vi "UHR-Fleezers Control (fpga) - 10.8c.vi"() -> ()   [LabVIEW 2014]
doc: "UHR-Fleezers Instrument Control Code (fpga)"
uses:
  <vilib>/eio/EIONode/EIONode.xnode
  <vilib>/eio/EIOMethodNode/EIOMethodNode.xnode
  <vilib>/rvi/DataTransferAndStorage/Container/XNode/niFpgaContainer.xnode
  <vilib>/Platform/TimedLoop/XDataNode/XDataNode.xnode
  <vilib>/Platform/TimedLoop/XDataNode/nitl_modes.ctl
  <vilib>/Platform/TimedLoop/XDataNode/XDNodeRunTimeDep.lvlib
  <vilib>/Platform/TimedLoop/XDataNode/wakeup.ctl
  <vilib>/Platform/TimedLoop/XDataNode/timing_clust.ctl
  <vilib>/addons/control/pid/fpga.llb/XNode/niFpgaPID.xnode
  <vilib>/rvi/eio/common/nirviEmuTemplateMethod_errors.vi
  <vilib>/rvi/interface/RandomDataEmulation/nirviRandomDataFpgaReadWriteTemplate.vi
panel:
  in  "Connector0/AO6":i16
  in  "Tab Control":T1(tab)=enum."Force FB"
  in  "Trap Pos to FIFO":bool
  in  "AI1 Sets to FIFO":T2={"Set 1"=TRUE, "Set 2"=TRUE, "Set 3"=FALSE}
  in  "N of AI1 Int Acq Sets":i16=2 min=1 max=3 step=1
  out "AI Late Counter":u8
  in  "ai count":u16=400
  in  "+ phase":bool
  in  "Phase count adjustment":i16
  out "Relative phase":i16
  in  "AI to FIFO":bool
  out "BD1 Frequency Out 1":u64
  out "BD1 Frequency Out 2":u64
  out "Trap Pos FIFO Timeout":u16
  out "Trap AI FIFO Timeout":u16
  in  "Trap FIFO Set Timeout":i32
  in  "Tab Control 2":T3(tab)
  out "Wiggling 2":bool
  in  "Abort wiggle 2":bool
  in  "Wiggle amp 2":u64
  in  "Wiggle freq 2 (Hz)":fxp<+/-,16,16>
  in  "Wiggle trap 2":bool
  out "Wiggling 1":bool
  in  "Abort wiggle 1":bool
  in  "Wiggle trap 1":bool
  in  "Wiggle amp 1":u64
  in  "Wiggle freq 1 (Hz)":fxp<+/-,16,16>
  in  "Swap F1 and F2":bool
  in  "Freq or Amp switch first":bool=TRUE
  in  "Cont. Scan":bool
  in  "Abort scan":bool
  in  "Cycles per step":u64
  in  "Scan BD":bool
  in  "Number of scans":u16
  in  "Scan steps":u64
  in  "Scan freq.  increment":i64
  out "Scanning":bool
  in  "Start scan":bool
  in  "OSK Bd 1":bool
  in  "Reset Bd 1":bool
  in  "RD":bool
  in  "PMODE":bool
  in  "OSK Bd 2":bool
  in  "Reset Bd 2":bool
  in  "Direct RF Box \nCommunication":bool
  in  "Data BD 2":u8 format="%08b"
  in  "Data BD 1":u8 format="%08b"
  in  "Address":u8 format="%02x"
  in  "Update Data":bool
  in  "FPGA Controls\n RF Box":bool
  in  "Number Interlace Cycles":u8=2 min=1 max=3
  in  "Interlace Off Parameters":u8=1 min=1 max=3
  in  "Interlace ON/OFF":bool
  out "DIO Relative phase":i16
  in  "Phase count adjustment (DIO)":i16
  in  "+ phase (DIO)":bool
  out "DIO Late Counter":u8
  in  "DIO count 1 (ticks)":u16=400
  in  "DIO count 2 (ticks)":u16=400
  in  "DIO count 3 (ticks)":u16=400
  out "AI2 Y Sum Set 2":i16
  out "AI2 Y Sum Set 1":i16
  in  "FB Gains Set 1":T4={"proportional gain (Kc)"=10, "integral gain (Kc*Ts/Ti)"=5, "derivative gain (Kc*Td/Ts)"=0}
  in  "FB Setpoint Set 1":i16 min=0 step=1
  in  "FB Reset Set 1":bool
  in  "FB On/Off Set 1":bool
  in  "FB Reset Set 2":bool
  in  "FB On/Off Set 2":bool
  in  "FB Setpoint Set 2":i16 min=0 step=1
  in  "FB Gains Set 2":T4={"proportional gain (Kc)"=10, "integral gain (Kc*Ts/Ti)"=5, "derivative gain (Kc*Td/Ts)"=0}
  in  "FB output range 2":cluster{"output high":i16, "output low":i16}={"output high"=3000, "output low"=0}
  in  "FB output range 1":cluster{"output high":i16, "output low":i16}={"output high"=3000, "output low"=0}
  out "Scan I":u64
  in  "Amp switch delay":u16=5
  in  "Freq switch delay":u16
  in  "BD 2 Amplitude 1":u16
  in  "BD 1 Amplitude 1":u16
  in  "BD 2 Frequency 1":u64
  in  "BD 1 Frequency 1":u64
  in  "BD 2 Amplitude 2":u16
  in  "BD 1 Amplitude 2":u16
  in  "BD 2 Frequency 2":u64
  in  "BD 1 Frequency 2":u64
  in  "BD 2 Amplitude 3":u16
  in  "BD 1 Amplitude 3":u16
  in  "BD 2 Frequency 3":u64
  in  "BD 1 Frequency 3":u64
  in  "Negate Diff?":bool
  in  "Diff FB Measurement?":bool
  in  "FB Trig Integrate":u32=1
  out "TTrig?":bool
  in  "TTrig Negate Pos":bool=TRUE
  out "Trap Pos FB Int Signal":fxp<+/-,24,9> format="%.18g"
  out "Trap Pos FB Int-Norm Signal":fxp<+/-,16,1> format="%.16g"
  in  "FPGA TTrig Thresh":i64
  in  "FPGA Trap Trig":bool
  out "Trap Pos FB Action":i64
  in  "Trap Pos. FB Offset Factor":i64
  in  "Trap Pos. FB Mult Factor":i64=2
  in  "Trap Pos. FB Range":T5={"output high"=0.999969482421875, "output low"=-1.0}
  in  "Trap Pos. FB Gains":T6={"proportional gain (Kc)"=0.0, "integral gain (Kc*Ts/Ti)"=10.0, "derivative gain (Kc*Td/Ts)"=0.0} {"proportional gain (Kc)" format="%.11g"; "integral gain (Kc*Ts/Ti)" format="%.11g"; "derivative gain (Kc*Td/Ts)" format="%.11g"}
  in  "Trap Pos. FB Reset":bool
  in  "Trap Pos FB Monitor T1 or T2":bool
  in  "AI1 X Scale":u16
  in  "Trap Pos FB Int Count":u16=100
  in  "Trap Pos FB Negate Action":bool
  out "AI1 X Set 2":fxp<+/-,16,1>
  out "AI1 X Set 1":fxp<+/-,16,1>
  in  "Trap Pos. FB SP":fxp<+/-,16,1>
  in  "Force feedback":bool
  out "TTrig Sig":i64
  out "TTrig Fin Thresh":i64
  out "Numeric":i32
  out "AO2 2":i16
  out "AO1 2":i16
  in  "1D or 2D Scan?":bool
  in  "Abort scan (MCL)":bool
  in  "MCL Scan Axis":bool
  in  "Cont. Scan (MCL)":bool
  out "Scan I (MCL)":u64
  in  "Number of scans (MCL)":u16
  out "Scanning MCL":bool
  in  "Scan steps (MCL)":u64
  in  "Cycles per step (MCL)":u64
  in  "Scan freq.  increment (MCL)":i16
  in  "Start scan (MCL)":bool
  in  "AO2":i16
  in  "AO1":i16
  out "MCL Late Counter":u8
  in  "MCL count":u32=800
  out "MCL Relative Phase":i16
  in  "Phase count adjustment (MCL)":i16
  in  "+ phase (MCL)":bool
  in  "APD Gate Operating Mode":u8 max=2 step=1
  in  "Invert APD Gate":bool
  in  "APD Gate OFF Count":u16=100
  in  "APD Gate ON Count":u16=300
  out "APD 1 Gate Late Counter":u8
  out "APD 1 Gate Relative Phase":i16
  in  "Phase count adjustment (APD 1 Gate)":i16
  in  "+ phase (APD 1 Gate)":bool
  out "APD 2 Counts 0":u32
  out "APD 2 Counts 1":u32
  out "APD 1 Counts 0":u32
  out "APD 1 Counts 1":u32
  out "APD 1 out state":bool
  in  "APD 2 AO scale factor":i16=1
  in  "APD 1 AO scale factor":i16=1
  in  "APD to FIFO":bool
  in  "APD Acq Rate Count":u32=20000000
  out "APD Acq Late Counter":u8
  out "APD Acq Relative Phase":i16
  in  "Phase Count Adjustment (APD Acq)":i16
  in  "+ phase (APD Acq)":bool
  in  "Phase count adjustment (APD 2 Gate)":i16
  out "APD 2 Gate Late Counter":u8
  out "APD 2 Gate Relative Phase":i16
  in  "+ phase (APD 2 Gate)":bool
  out "APD 2 out state":bool
  out "APD 1 Int Gate":bool
  out "APD 2 Int Gate":bool
  in  "Green Filter Flipper":bool
  out "Green FB Signals":T7
  in  "Green FB Count":u16=1200
  out "Green Late Counter":u8
  out "Green FB Relative Phase":i16
  in  "Phase count adjustment (Green FB)":i16=10
  in  "+ phase (Green FB)":bool
  out "Green FB Sum":i16
  in  "Green int current ON count adj":u16=150
  in  "Current Out":u16=30000
  in  "Green FB On/Off":bool
  in  "Green FB Setpoint":i16=250 min=0 step=1
  in  "Green FB Gains":T4={"proportional gain (Kc)"=10, "integral gain (Kc*Ts/Ti)"=5, "derivative gain (Kc*Td/Ts)"=0}
  in  "Green FB Reset":bool
  in  "Operating Mode 2":u8=2 max=2 step=1
  in  "Invert GI 2":bool
  in  "Green interlace OFF count 2":u16=900
  in  "Green interlace ON count 2":u16=300
  out "GI Late Counter 2":u8
  out "GI Relative phase 2":i16
  in  "Phase count adjustment (GI) 2":i16=20
  in  "+ phase (GI) 2":bool
  in  "Green interlace OFF count":u16=100
  out "GI Relative phase":i16
  in  "Phase count adjustment (GI)":i16
  in  "+ phase (GI)":bool
  in  "Green interlace ON count":u16=300
  out "GI Late Counter":u8
  in  "Invert GI":bool
  in  "Operating Mode":u8 max=2 step=1
  in  "Invert RI 2":bool
  in  "Invert RI":bool
  in  "Phase count adjustment (RI)":i16
  in  "+ phase (RI)":bool
  in  "RI OFF count":u16
  in  "RI ON count":u16
  in  "RI Current Out":u16
  in  "RI operating mode 2":u8
  in  "Red operating mode":u8
  out "RI late counter":u8
  out "RI relative phase":i16
  in  "Chassis2/Mod4/AO1":u16
  # "Only one of these can be on\nat a time:"
  # "Raster Scan AOD"
  # "1 (X)"
  # "2 (Y)"
  # "IR Intensity Feedback (RF BD 1)"
  # "FB Triggering Excitation Laser"
  # "AO1 (Y)"
  # "2D"
  # "1D"
  # "AO2 (X)"
  # "APD AO for aligning"
  # "Detection Loop"
  # "Green fluorescent laser digital gate interlacing loop"
  # "0 Forced ON\n1 Forced OFF\n2 Interlacing"
  # "Red fluorescent laser digital gate interlacing loop"
  # "0 Forced ON\n1 Forced OFF\n2 Interlacing"
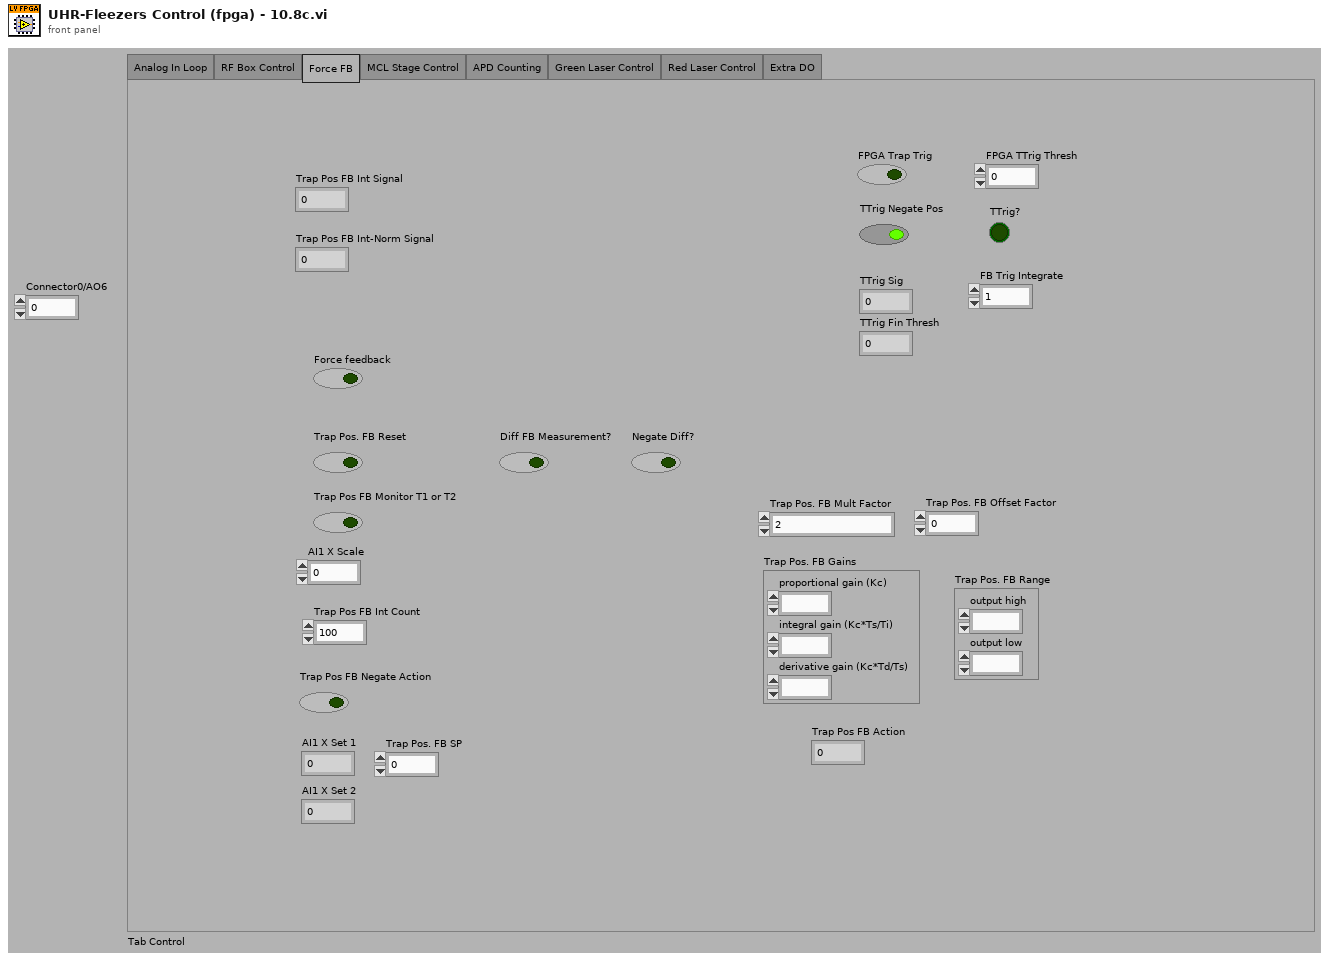
[diagram p1: front panel]
types:
  T1 = enum32{"Analog In Loop", "RF Box Control", "Force FB", "MCL Stage Control", "APD Counting", "Green Laser Control", "Red Laser Control", "Extra DO"}
  T2 = cluster{"Set 1":bool, "Set 2":bool, "Set 3":bool}
  T3 = enum32{"Controls", "Interlacing Frequency and Amplitude Values"}
  T4 = cluster{"proportional gain (Kc)":i16, "integral gain (Kc*Ts/Ti)":i16, "derivative gain (Kc*Td/Ts)":i16}
  T5 = cluster{"output high":fxp<+/-,16,1>, "output low":fxp<+/-,16,1>}
  T6 = cluster{"proportional gain (Kc)":fxp<+/-,16,8>, "integral gain (Kc*Ts/Ti)":fxp<+/-,16,8>, "derivative gain (Kc*Td/Ts)":fxp<+/-,16,8>}
  T7 = cluster{"Green FB Ch 0":i16, "Green FB Ch 1":i16, "Green FB Ch 2":i16}
  T8 = typedef "XDNodeRunTimeDep.lvlib/timing_clust.ctl" = cluster{"Expected End [f-1]":u64, "Actual End [f-1]":u64, "Finished Late? [f-1]":bool, "Expected End [i-1]":u64, "Actual End [i-1]":u64, "Finished Late? [i-1]":bool, "Expected Start [i]":u64, "Actual Start [i]":u64, "Expected Start [f]":u64, "Actual Start [f]":u64, "Source Name":string, "Structure Name":string, "Period":i64, "Deadline":i64, "Offset":i64, "Start":i64, "Priority":i32, "Timeout":i32, "Mode":T9, "Wakeup Reason":T10, "Error":errorcluster, "Source Type":string, "Secondary Source Type":string, "Global End Time":u64, "Global Start Time":u64, "Frame Duration":u64, "Iteration Duration":u64, "Assigned CPU":i32, "I/O Scan Engine Mode":u32}
  T9 = typedef "XDNodeRunTimeDep.lvlib/nitl_modes.ctl" = enum32{"No Change", "Process missed periods, maintain original phase", "Discard missed periods, maintain original phase", "Process missed periods, ignore original phase", "Discard missed periods, ignore original phase"}
  T10 = typedef "XDNodeRunTimeDep.lvlib/wakeup.ctl" = enum32{"Normal", "Aborted", "Asynchronous wakeup", "Timing source error", "Timed loop error", "Timeout"}
  T11 = cluster{"Chassis2/Mod1/AI0":void, "Chassis2/Mod1/AI1":void, "Chassis2/Mod1/AI2":void}
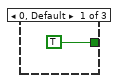
[diagram p2: hidden frame]
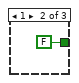
[diagram p3: hidden frame]
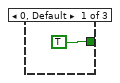
[diagram p4: hidden frame]
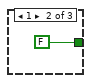
[diagram p5: hidden frame]
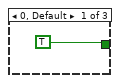
[diagram p6: hidden frame]
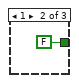
[diagram p7: hidden frame]
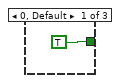
[diagram p9: hidden frame]
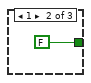
[diagram p10: hidden frame]
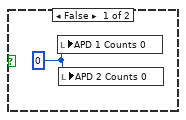
[diagram p11: hidden frame]
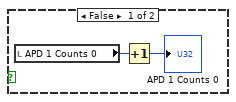
[diagram p14: hidden frame]
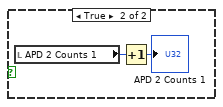
[diagram p16: hidden frame]
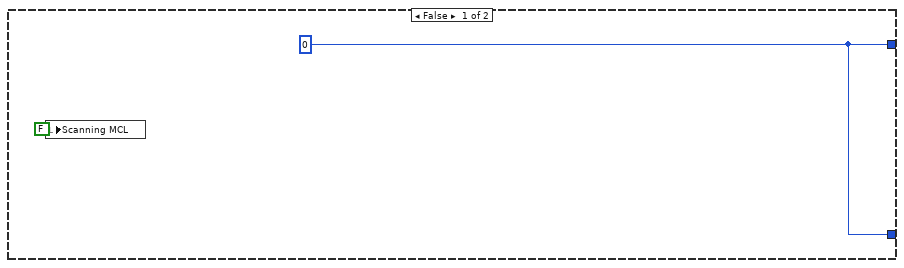
[diagram p17: hidden frame]
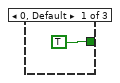
[diagram p18: hidden frame]
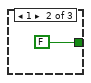
[diagram p19: hidden frame]
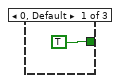
[diagram p20: hidden frame]
diagram:
  w1 = u16 0
  w4 = FALSE
  w2 = FALSE
  # "633 nm red excitation laser interlacing (DO to IA 633 nm AOM ME amp)."
  # "The APD Int Gate is here so the FPGA will do the integration only when the APD gate is \"ON\" (though we will leave the APD continuously ON now). This was added because the actual APD gating (via the hardware) was giving false signals. -KW"
  # "timing array current index"
  # "timing array"
  # "timing counter (phase adjusted here)"
  # "late counter"
  n1 = flat-sequence "FPGA initialization to do before running any of the loops" {
    tunnel: [u16 0 ("DIO count 3 (ticks)")] -> w3
    tunnel: [w10] -> _
    frame #0 {
      # "Start up expansion chassis early\nto avoid delays later"
      # "This pin controls udclk on the RF boards.\nWhen initially configuring the boards, this pin needs to be\nconfigured as a high impedance input.  Later it will be switched\nto an output."
      # "Initial setting of DIO data and \naddress to low (before reset).  \nThis needs to happen before the other\ncontrol method loops execute."
      n2 = xnode "FPGA I/O Node"("Chassis2/Mod4/AO0"=u16 0) -> ("Chassis2/Mod1/AI0"=w10)  [unwired: 2 in, 2 out]
      n3 = xnode "FPGA I/O Method Node"("Enable"=FALSE) -> ()  [unwired: 1 in, 1 out]
      n4 = xnode "FPGA I/O Node"("Connector1/DIO0"=FALSE, "Connector1/DIO1"=FALSE, "Connector1/DIO2"=FALSE, "Connector1/DIO3"=FALSE, "Connector1/DIO4"=FALSE, "Connector1/DIO5"=FALSE, "Connector1/DIO6"=FALSE, "Connector1/DIO7"=FALSE, "Connector1/DIO8"=FALSE, "Connector1/DIO9"=FALSE, "Connector1/DIO10"=FALSE, "Connector1/DIO11"=FALSE, "Connector1/DIO12"=FALSE, "Connector1/DIO13"=FALSE, "Connector1/DIO15"=FALSE, "Connector1/DIO20"=FALSE, "Connector1/DIO21"=FALSE, "Connector1/DIO22"=FALSE, "Connector1/DIO23"=FALSE, "Connector1/DIO24"=FALSE, "Connector1/DIO25"=FALSE, "Connector1/DIO26"=FALSE, "Connector1/DIO27"=FALSE, "Connector1/DIO14"=FALSE) -> ()  [unwired: 24 in, 24 out]
    }
  }
  n5 = local read "AO1"() -> (w8:i16)
  n6 = local read "AO2"() -> (w7:i16)
  n7 = node-c288() -> (w6:T8)  [unwired: 1 in]
  n8 = while "APD 1 Counter" {
    tunnel: w3 -> [_]
    stop <- FALSE stop-if-true
    n9 = flat-sequence {
      frame #0 {
        n10 = xnode "FPGA I/O Method Node"("FPGA I/O In"=refnum<k21> "Connector0/DIO0" ("APD 1 DO"), "Timeout"=-1) -> ()  [unwired: 2 out]
      }
      frame #1 {
        n11 = local read "APD 1 Int Gate"() -> (w41:bool)
        n12 = case shown="True" w41 {
          frame False {
          }
          frame True {
            n13 = local read "APD 1 out state"() -> (w42:bool)
            n14 = case shown="True" w42 {
              frame False {
                n15 = local read "APD 1 Counts 0"() -> (w44:u32)
                n16 = Increment(x=w44) -> (x+1=→"APD 1 Counts 0":u32)
              }
              frame True {
                n17 = local read "APD 1 Counts 1"() -> (w46:u32)
                n18 = Increment(x=w46) -> (x+1=→"APD 1 Counts 1":u32)
              }
            }
          }
        }
      }
    }
  }
  n19 = while "APD 2 Counter" {
    tunnel: w3 -> [_]
    stop <- FALSE stop-if-true
    n20 = flat-sequence {
      frame #0 {
        n21 = xnode "FPGA I/O Method Node"("FPGA I/O In"=refnum<k21> "Connector0/DIO1" ("APD 2 DO"), "Timeout"=-1) -> ()  [unwired: 2 out]
      }
      frame #1 {
        n22 = local read "APD 2 Int Gate"() -> (w50:bool)
        n23 = case shown="True" w50 {
          frame False {
          }
          frame True {
            n24 = local read "APD 2 out state"() -> (w51:bool)
            n25 = case shown="False" w51 {
              frame False {
                n26 = local read "APD 2 Counts 0"() -> (w53:u32)
                n27 = Increment(x=w53) -> (x+1=→"APD 2 Counts 0":u32)
              }
              frame True {
                n28 = local read "APD 2 Counts 1"() -> (w55:u32)
                n29 = Increment(x=w55) -> (x+1=→"APD 2 Counts 1":u32)
              }
            }
          }
        }
      }
    }
  }
  n30 = while "APD 2 Gating" {
    shift-right: [w59] -> _
    shift-left: w3 -> [w64]
    shift-right: [w58] -> _
    shift-left: w4 -> [w56]
    stop <- FALSE stop-if-true
    n31 = flat-sequence {
      tunnel: w64 -> [w67]
      tunnel: [w68] -> w62
      tunnel: [w67] -> w60
      tunnel: [w66] -> w57
      tunnel: w56 -> [w66]
      tunnel: [w71] -> w63
      tunnel: w62 -> [w71]
      tunnel: [w70] -> w61
      tunnel: w60 -> [w70]
      tunnel: w57 -> [w69]
      tunnel: [w89] -> w59
      tunnel: w63 -> [w100]
      tunnel: w61 -> [w98]
      tunnel: [w93] -> w58
      frame #0 {
        n32 = call "Loop Timer8"("Count(Ticks)"=w67) -> ("Tick Count(Ticks)"=w68:u16)
      }
      frame #1 {
        # "(need 4 channels/APD)"
        n33 = xnode "FPGA I/O Node"("Connector0/DIO8"=w69, "Connector0/DIO9"=w69, "Connector0/DIO10"=w69, "Connector0/DIO11"=w69) -> ()  [unwired: 4 in, 4 out]
        "APD 2 Int Gate" <- w69
      }
      frame #2 {
        n34 = local read "APD Gate ON Count"() -> (w82:u16)
        n35 = local read "APD Gate OFF Count"() -> (w81:u16)
        n36 = feedback #1(TRUE) -> (w95:bool)
        n37 = feedback-in #2(w100) -> ()
        n38 = feedback #2(w100) -> (w83:u16)
        n39 = Not(x=w95) -> (.not. x?=w92:bool)
        n40 = feedback-in #1(w92) -> ()
        n41 = Subtract(x=w100, y=w83) -> (x-y=w99:u16)
        n42 = Select(t=w82, s=w92, f=w81) -> (s? t:f=w97:u16)
        n43 = Subtract(x=w99, y=w98) -> (x-y=w74:u16)
        n44 = Subtract(x=w97, y=w74) -> (x-y=w88:u16)
        n45 = Number To Boolean Array(number=w74) -> (Boolean array=w73:bool[])
        n46 = Or Array Elements(Boolean array=w73) -> (logical OR=w72:bool)
        n47 = Boolean To (0,1)(Boolean="+ phase (APD 2 Gate)") -> (0, 1=w86:i16)
        n48 = Multiply(x=w86, y="Phase count adjustment (APD 2 Gate)") -> (x*y=w84:i16)
        n49 = Boolean To (0,1)(Boolean=w72) -> (0, 1=w79:i16)
        n50 = Add(x=w88, y=w84) -> (x+y=w89:u16)
        n51 = To Unsigned Byte Integer(number=w79) -> (unsigned 8bit integer=w76:u8)
        n52 = feedback #3(i16 0) -> (w91:i16)
        n53 = Subtract(x=w91, y=w84) -> (x-y=w90:i16)
        "APD 2 Gate Relative Phase" <- w90
        n54 = feedback-in #3(w90) -> ()
        n55 = feedback #4(u8 0) -> (w77:u8)
        n56 = Add(x=w76, y=w77) -> (x+y=w75:u8)
        "APD 2 Gate Late Counter" <- w75
        n57 = feedback-in #4(w75) -> ()
        n58 = local read "APD Gate Operating Mode"() -> (w80:u8)
        n59 = case shown="2" w80 {
          tunnel: [TRUE FALSE w106] -> w93
          tunnel: w95 -> [_ _ w104]
          frame 0, Default {
          }
          frame 1 {
          }
          frame 2 {
            n60 = local read "Invert APD Gate"() -> (w103:bool)
            n61 = Not(x=w104) -> (.not. x?=w105:bool)
            n62 = Select(t=w105, s=w103, f=w104) -> (s? t:f=w106:bool)
          }
        }
      }
    }
  }
  n63 = while "APD 1 Gating" {
    shift-right: [w110] -> _
    shift-left: w3 -> [w115]
    shift-right: [w109] -> _
    shift-left: w4 -> [w107]
    stop <- FALSE stop-if-true
    n64 = flat-sequence {
      tunnel: w115 -> [w118]
      tunnel: [w119] -> w113
      tunnel: [w118] -> w111
      tunnel: [w117] -> w108
      tunnel: w107 -> [w117]
      tunnel: [w122] -> w114
      tunnel: w113 -> [w122]
      tunnel: [w121] -> w112
      tunnel: w111 -> [w121]
      tunnel: w108 -> [w120]
      tunnel: [w136] -> w110
      tunnel: w114 -> [w151]
      tunnel: w112 -> [w148]
      tunnel: [w140] -> w109
      frame #0 {
        n65 = call "Loop Timer7"("Count(Ticks)"=w118) -> ("Tick Count(Ticks)"=w119:u16)
      }
      frame #1 {
        # "(need 4 channels/APD)"
        n66 = xnode "FPGA I/O Node"("Connector0/DIO4"=w120, "Connector0/DIO5"=w120, "Connector0/DIO6"=w120, "Connector0/DIO7"=w120) -> ()  [unwired: 4 in, 4 out]
        "APD 1 Int Gate" <- w120
      }
      frame #2 {
        n67 = feedback #5(TRUE) -> (w143:bool)
        n68 = feedback-in #6(w151) -> ()
        n69 = feedback #6(w151) -> (w150:u16)
        n70 = Not(x=w143) -> (.not. x?=w139:bool)
        n71 = feedback-in #5(w139) -> ()
        n72 = Subtract(x=w151, y=w150) -> (x-y=w149:u16)
        n73 = Select(t="APD Gate ON Count", s=w139, f="APD Gate OFF Count") -> (s? t:f=w145:u16)
        n74 = Subtract(x=w149, y=w148) -> (x-y=w124:u16)
        n75 = Subtract(x=w145, y=w124) -> (x-y=w135:u16)
        n76 = Number To Boolean Array(number=w124) -> (Boolean array=w125:bool[])
        n77 = Or Array Elements(Boolean array=w125) -> (logical OR=w123:bool)
        n78 = Boolean To (0,1)(Boolean="+ phase (APD 1 Gate)") -> (0, 1=w133:i16)
        n79 = Boolean To (0,1)(Boolean=w123) -> (0, 1=w130:i16)
        n80 = Multiply(x=w133, y="Phase count adjustment (APD 1 Gate)") -> (x*y=w131:i16)
        n81 = To Unsigned Byte Integer(number=w130) -> (unsigned 8bit integer=w127:u8)
        n82 = Add(x=w135, y=w131) -> (x+y=w136:u16)
        n83 = feedback #7(i16 0) -> (w138:i16)
        n84 = Subtract(x=w138, y=w131) -> (x-y=w137:i16)
        "APD 1 Gate Relative Phase" <- w137
        n85 = feedback-in #7(w137) -> ()
        n86 = feedback #8(u8 0) -> (w128:u8)
        n87 = Add(x=w127, y=w128) -> (x+y=w126:u8)
        "APD 1 Gate Late Counter" <- w126
        n88 = feedback-in #8(w126) -> ()
        n89 = case shown="2" "APD Gate Operating Mode" {
          tunnel: [TRUE FALSE w157] -> w140
          tunnel: w143 -> [_ _ w154]
          frame 0, Default {
          }
          frame 1 {
          }
          frame 2 {
            n90 = Not(x=w154) -> (.not. x?=w156:bool)
            n91 = Select(t=w156, s="Invert APD Gate", f=w154) -> (s? t:f=w157:bool)
          }
        }
      }
    }
  }
  n92 = timed-loop "RF box board DIO control: control bits" {
    timing: w6 -> [_]
    timing-out: [_] -> w5
    tunnel: [w158] -> _
    tunnel: w3 -> [w158]
    stop <- FALSE stop-if-true
    n93 = xnode "FPGA I/O Node"("Connector1/DIO16"="RD", "Connector1/DIO17"="PMODE", "Connector1/DIO18"="OSK Bd 1", "Connector1/DIO19"="Reset Bd 1", "Connector1/DIO28"="OSK Bd 2", "Connector1/DIO29"="Reset Bd 2") -> ()  [unwired: 6 in, 6 out]
  }
  n94 = while "532 nm green excitation laser interlacing (DO to IA 532 nm AOM ME amp)." {
    shift-right: [w171] -> _
    shift-left: w3 -> [w176]
    shift-right: [w170] -> _
    shift-left: w2 -> [w168]
    stop <- FALSE stop-if-true
    n95 = flat-sequence {
      tunnel: w176 -> [w179]
      tunnel: [w180] -> w174
      tunnel: [w179] -> w172
      tunnel: [w178] -> w169
      tunnel: w168 -> [w178]
      tunnel: [w183] -> w175
      tunnel: w174 -> [w183]
      tunnel: [w182] -> w173
      tunnel: w172 -> [w182]
      tunnel: w169 -> [w181]
      tunnel: [w192] -> w171
      tunnel: w175 -> [w212]
      tunnel: w173 -> [w209]
      tunnel: [w201] -> w170
      frame #0 {
        n96 = call "Loop Timer4"("Count(Ticks)"=w179) -> ("Tick Count(Ticks)"=w180:u16)
      }
      frame #1 {
        n97 = xnode "FPGA I/O Node"("Connector1/DIO37"=w181, "Connector1/DIO38"=w181, "Connector1/DIO39"=w181) -> ()  [unwired: 3 in, 3 out]
      }
      frame #2 {
        n98 = feedback-in #9(w212) -> ()
        n99 = feedback #9(w212) -> (w211:u16)
        n100 = Subtract(x=w212, y=w211) -> (x-y=w210:u16)
        n101 = Subtract(x=w210, y=w209) -> (x-y=w185:u16)
        n102 = Number To Boolean Array(number=w185) -> (Boolean array=w186:bool[])
        n103 = Or Array Elements(Boolean array=w186) -> (logical OR=w184:bool)
        n104 = Boolean To (0,1)(Boolean="+ phase (GI)") -> (0, 1=w197:i16)
        n105 = Multiply(x=w197, y="Phase count adjustment (GI)") -> (x*y=w194:i16)
        n106 = Boolean To (0,1)(Boolean=w184) -> (0, 1=w191:i16)
        n107 = To Unsigned Byte Integer(number=w191) -> (unsigned 8bit integer=w188:u8)
        n108 = feedback #10(i16 0) -> (w195:i16)
        n109 = feedback #11(u8 0) -> (w189:u8)
        n110 = Add(x=w188, y=w189) -> (x+y=w187:u8)
        "GI Late Counter" <- w187
        n111 = feedback-in #11(w187) -> ()
        n112 = Subtract(x=w195, y=w194) -> (x-y=w193:i16)
        "GI Relative phase" <- w193
        n113 = feedback-in #10(w193) -> ()
        n114 = feedback #12(TRUE) -> (w204:bool)
        n115 = case shown="2" "Operating Mode" {
          tunnel: [TRUE FALSE w218] -> w201
          tunnel: w204 -> [_ _ w215]
          frame 0, Default {
          }
          frame 1 {
          }
          frame 2 {
            n116 = Not(x=w215) -> (.not. x?=w217:bool)
            n117 = Select(t=w217, s="Invert GI", f=w215) -> (s? t:f=w218:bool)
          }
        }
        n118 = Not(x=w204) -> (.not. x?=w200:bool)
        n119 = Select(t="Green interlace ON count", s=w200, f="Green interlace OFF count") -> (s? t:f=w206:u16)
        n120 = Subtract(x=w206, y=w185) -> (x-y=w198:u16)
        n121 = Add(x=w198, y=w194) -> (x+y=w192:u16)
        n122 = feedback-in #12(w200) -> ()
      }
    }
  }
  n123 = while "Green and red excitation laser interlacing (Current AO to IA 532 nm AOM ME amp)." {
    shift-right: [w227] -> _
    shift-left: w3 -> [w230]
    shift-right: [w224] -> _
    shift-left: w1 -> [w222]
    shift-right: [w219] -> _
    shift-left: w1 -> [w221]
    stop <- FALSE stop-if-true
    n124 = flat-sequence {
      tunnel: w230 -> [w234]
      tunnel: [w235] -> w229
      tunnel: [w234] -> w228
      tunnel: [w233] -> w223
      tunnel: w222 -> [w233]
      tunnel: w221 -> [w232]
      tunnel: [w232] -> w220
      tunnel: [w239] -> w226
      tunnel: w229 -> [w239]
      tunnel: [w238] -> w225
      tunnel: w228 -> [w238]
      tunnel: w223 -> [w237]
      tunnel: w220 -> [w236]
      tunnel: [w256] -> w227
      tunnel: [w273] -> w224
      tunnel: w226 -> [w240]
      tunnel: w225 -> [w282]
      tunnel: [w242] -> w219
      frame #0 {
        n125 = call "Loop Timer10"("Count(Ticks)"=w234) -> ("Tick Count(Ticks)"=w235:u16)
      }
      frame #1 {
        n126 = xnode "FPGA I/O Node"("Chassis2/Mod4/AO0"=w237, "Chassis2/Mod4/AO1"=w236) -> ()  [unwired: 2 in, 2 out]
      }
      frame #2 {
        # "Design note (Comstock lab):\n\nThese two laser controls are in the same loop\nbecause the expansion current AI cannot separately\ntime the outputs fast enough for us.  Apparently\nit is because of communication time between the\nexpansion card and the fpga.\n\nSo the two analog control signals have the same timing\nand profile, but independent amplitudes to independently\ncontrol the intensity and feedback for each laser."
        n127 = feedback #13(TRUE) -> (w241:bool)
        n128 = Subtract(x="Green interlace OFF count 2", y="Green int current ON count adj") -> (x-y=w265:u16)
        n129 = Not(x=w241) -> (.not. x?=w275:bool)
        n130 = feedback-in #13(w275) -> ()
        n131 = feedback-in #14(w240) -> ()
        n132 = feedback #14(w240) -> (w284:u16)
        n133 = Add(x="Green int current ON count adj", y="Green interlace ON count 2") -> (x+y=w266:u16)
        n134 = Subtract(x=w240, y=w284) -> (x-y=w283:u16)
        n135 = Select(t=w266, s=w275, f=w265) -> (s? t:f=w279:u16)
        n136 = Subtract(x=w283, y=w282) -> (x-y=w249:u16)
        n137 = case shown="2" "RI operating mode 2" {
          tunnel: [TRUE FALSE w287] -> w246
          tunnel: w241 -> [_ _ w289]
          frame 0, Default {
          }
          frame 1 {
          }
          frame 2 {
            n138 = Not(x=w289) -> (.not. x?=w288:bool)
            n139 = Select(t=w288, s="Invert RI 2", f=w289) -> (s? t:f=w287:bool)
          }
        }
        n140 = case shown="2" "Operating Mode 2" {
          tunnel: [TRUE FALSE w307] -> w267
          tunnel: w241 -> [_ _ w304]
          frame 0, Default {
          }
          frame 1 {
          }
          frame 2 {
            n141 = Not(x=w304) -> (.not. x?=w306:bool)
            n142 = Select(t=w306, s="Invert GI 2", f=w304) -> (s? t:f=w307:bool)
          }
        }
        n143 = Subtract(x=w279, y=w249) -> (x-y=w260:u16)
        n144 = Number To Boolean Array(number=w249) -> (Boolean array=w250:bool[])
        n145 = Boolean To (0,1)(Boolean="+ phase (GI) 2") -> (0, 1=w262:i16)
        n146 = Or Array Elements(Boolean array=w250) -> (logical OR=w248:bool)
        n147 = Boolean To (0,1)(Boolean=w248) -> (0, 1=w255:i16)
        n148 = Multiply(x=w262, y="Phase count adjustment (GI) 2") -> (x*y=w258:i16)
        n149 = To Unsigned Byte Integer(number=w255) -> (unsigned 8bit integer=w251:u8)
        n150 = Add(x=w260, y=w258) -> (x+y=w256:u16)
        n151 = feedback #15(u8 0) -> (w253:u8)
        n152 = Add(x=w251, y=w253) -> (x+y=w252:u8)
        "GI Late Counter 2" <- w252
        n153 = feedback-in #15(w252) -> ()
        n154 = feedback #16(i16 0) -> (w259:i16)
        n155 = Subtract(x=w259, y=w258) -> (x-y=w257:i16)
        "GI Relative phase 2" <- w257
        n156 = feedback-in #16(w257) -> ()
        n157 = And(x=w267, y="Green FB On/Off") -> (x .and. y?=w268:bool)
        n158 = case shown="True" w268 {
          tunnel: "Current Out" -> [w291 _]
          tunnel: [w291 w296] -> w272
          frame False {
          }
          frame True {
            n159 = local read "Green FB Sum"() -> (w292:i16)
            n160 = call "Slower PID.vi"("process variable"=w292, "reset?"="Green FB Reset", "setpoint"="Green FB Setpoint", "PID gains (x 2^8)"="Green FB Gains", "output range"=cluster{"output high":i16, "output low":i16} {"output high"=32767, "output low"=-32768} ("Green FB output range")) -> ("output"=w300:i16)  [unwired: 10 out]
            n161 = To Long Integer(number=w300) -> (32bit integer=w293:i32)
            n162 = Add(x=w293, y=32768) -> (x+y=w295:i32)
            n163 = To Unsigned Word Integer(number=w295) -> (unsigned 16bit integer=w296:u16)
          }
        }
        n164 = Boolean To (0,1)(Boolean=w246) -> (0, 1=w245:i16)
        n165 = Boolean To (0,1)(Boolean=w267) -> (0, 1=w274:i16)
        n166 = To Unsigned Word Integer(number=w274) -> (unsigned 16bit integer=w271:u16)
        n167 = To Unsigned Word Integer(number=w245) -> (unsigned 16bit integer=w244:u16)
        n168 = Multiply(x=w271, y=w272) -> (x*y=w273:u16)
        n169 = Multiply(x=w244, y="RI Current Out") -> (x*y=w242:u16)
      }
    }
  }
  n170 = while "Green excitation laser feedback measurement" {
    shift-right: [w308] -> _
    shift-left: w3 -> [w313]
    stop <- FALSE stop-if-true
    n171 = flat-sequence {
      tunnel: w313 -> [w315]
      tunnel: [w316] -> w311
      tunnel: [w315] -> w309
      tunnel: [w323] -> w312
      tunnel: w311 -> [w323]
      tunnel: [w322] -> w310
      tunnel: w309 -> [w322]
      tunnel: [w335] -> w308
      tunnel: w312 -> [w346]
      tunnel: w310 -> [w343]
      frame #0 {
        n172 = call "Loop Timer9"("Count(Ticks)"=w315) -> ("Tick Count(Ticks)"=w316:u16)
      }
      frame #1 {
        n173 = xnode "FPGA I/O Node"("Connector1/DIO35"=TRUE) -> ("Chassis2/Mod1/AI0"=w321, "Chassis2/Mod1/AI1"=w320, "Chassis2/Mod1/AI2"=w317)  [unwired: 4 in, 4 out]
        "Green FB Sum" <- w317
        n174 = Bundle("Chassis2/Mod1/AI0"=w321, "Chassis2/Mod1/AI1"=w320, "Chassis2/Mod1/AI2"=w317) -> (→"Green FB Signals":T11)  [unwired: 1 out]
      }
      frame #2 {
        n175 = feedback-in #17(w346) -> ()
        n176 = feedback #17(w346) -> (w345:u16)
        n177 = Subtract(x=w346, y=w345) -> (x-y=w344:u16)
        n178 = xnode "FPGA I/O Node"("Connector1/DIO35"=FALSE) -> ()  [unwired: 1 in, 1 out]
        n179 = Subtract(x=w344, y=w343) -> (x-y=w325:u16)
        n180 = Subtract(x="Green FB Count", y=w325) -> (x-y=w339:u16)
        n181 = Number To Boolean Array(number=w325) -> (Boolean array=w326:bool[])
        n182 = Or Array Elements(Boolean array=w326) -> (logical OR=w324:bool)
        n183 = Boolean To (0,1)(Boolean="+ phase (Green FB)") -> (0, 1=w337:i16)
        n184 = Boolean To (0,1)(Boolean=w324) -> (0, 1=w331:i16)
        n185 = Multiply(x=w337, y="Phase count adjustment (Green FB)") -> (x*y=w332:i16)
        n186 = Add(x=w339, y=w332) -> (x+y=w335:u16)
        n187 = To Unsigned Byte Integer(number=w331) -> (unsigned 8bit integer=w328:u8)
        n188 = feedback #18(i16 0) -> (w334:i16)
        n189 = Subtract(x=w334, y=w332) -> (x-y=w333:i16)
        "Green FB Relative Phase" <- w333
        n190 = feedback-in #18(w333) -> ()
        n191 = feedback #19(u8 0) -> (w329:u8)
        n192 = Add(x=w328, y=w329) -> (x+y=w327:u8)
        "Green Late Counter" <- w327
        n193 = feedback-in #19(w327) -> ()
      }
    }
  }
  n194 = while "Control Additional IO (Green laser flip mount)" {
    stop <- FALSE stop-if-true
    n195 = xnode "FPGA I/O Node"("Connector0/DIO3"="Green Filter Flipper", "Chassis2/Mod4/AO1"="Chassis2/Mod4/AO1", "Connector0/AO6"="Connector0/AO6") -> ()  [unwired: 3 in, 3 out]
    n196 = call "Loop Timer2"("Count(Ticks)"=u32 40000 ("Extra DO Counts")) -> ()  [unwired: 1 out]
  }
  n197 = while "DAQ AI set 1" {
    shift-right: [w352] -> _
    shift-left: w3 -> [w357]
    stop <- FALSE stop-if-true
    n198 = flat-sequence {
      tunnel: w357 -> [w367]
      tunnel: [w368] -> w355
      tunnel: [w367] -> w354
      tunnel: [w378] -> w365
      tunnel: [w377] -> w364
      tunnel: [w376] -> w363
      tunnel: [w375] -> w362
      tunnel: [w374] -> w361
      tunnel: [w373] -> w360
      tunnel: [w372] -> w359
      tunnel: [w371] -> w358
      tunnel: [w370] -> w356
      tunnel: w355 -> [w370]
      tunnel: w354 -> [w369]
      tunnel: [w369] -> w353
      tunnel: [w407] -> w352
      tunnel: w365 -> [w435]
      tunnel: w364 -> [w399]
      tunnel: w363 -> [w400]
      tunnel: w362 -> [w434]
      tunnel: w361 -> [w423]
      tunnel: w360 -> [w422]
      tunnel: w359 -> [w421]
      tunnel: w358 -> [w420]
      tunnel: w356 -> [w417]
      tunnel: w353 -> [w414]
      frame #0 {
        n199 = call "Loop Timer3"("Count(Ticks)"=w367) -> ("Tick Count(Ticks)"=w368:u16)
      }
      frame #1 {
        n200 = xnode "FPGA I/O Node"("Connector1/DIO31"=TRUE ("Connector1/DIO33")) -> ("Connector0/AI0"=w378, "Connector0/AI1"=w377, "Connector0/AI2"=w376, "Connector0/AI3"=w375, "Connector0/AI4"=w374, "Connector0/AI5"=w373, "Connector0/AI6"=w372, "Connector0/AI7"=w371)  [unwired: 9 in, 9 out]
      }
      frame #2 {
        w403 = FALSE ("AI to FIFO")
        # "Adjust phase after data acquired if button pressed"
        n201 = feedback #20(i16 1) -> (w427:i16)
        n202 = Increment(x=w427) -> (x+1=w433:i16)
        n203 = Scale By Power Of 2(n="AI1 X Scale", x=w399) -> (x*2^n=w397:dbl)
        n204 = Greater?(x=w433, y="N of AI1 Int Acq Sets") -> (0:w430:bool)
        n205 = Select(t=i16 1, s=w430, f=w433) -> (s? t:f=w432:i16)
        n206 = feedback-in #20(w432) -> ()
        n207 = Divide(x=w397, y=w400) -> (x/y=w396:fxp<+/-,16,1>)
        n208 = feedback #21(w403) -> (w401:bool)
        n209 = feedback #22(w403) -> (w419:bool)
        n210 = case shown="1, Default" w427 {
          tunnel: w400 -> [w457 w465 _]
          tunnel: "AI1 Sets to FIFO" -> [w461 w469 w475]
          tunnel: [w460 w468 w474] -> w424
          tunnel: ["AI to FIFO" w467 w473] -> w418
          tunnel: w419 -> [_ w467 w473]
          tunnel: ["Trap Pos to FIFO" w466 w472] -> w402
          tunnel: w401 -> [_ w466 w472]
          tunnel: w396 -> [w456 w464 _]
          tunnel: [w455 w462 FALSE] -> w383
          tunnel: [w454 w463 u64 0 ("BD1 Frequency Out 2")] -> w382
          frame 1, Default {
            n211 = Unbundle By Name(w461) -> ("Set 1"=w460:bool)
            n212 = local read "BD1 Frequency Out 1"() -> (w454:u64)
            n213 = Compound Arithmetic op=AND("Trap Pos to FIFO", w460, "AI to FIFO") -> (w455:bool)
            "AI2 Y Sum Set 1" <- w457
            "AI1 X Set 1" <- w456
          }
          frame 2 {
            n214 = Unbundle By Name(w469) -> ("Set 2"=w468:bool)
            n215 = local read "BD1 Frequency Out 2"() -> (w463:u64)
            n216 = Compound Arithmetic op=AND(w466, w468, w467) -> (w462:bool)
            "AI2 Y Sum Set 2" <- w465
            "AI1 X Set 2" <- w464
          }
          frame 3 {
            n217 = Unbundle By Name(w475) -> ("Set 3"=w474:bool)
          }
        }
        n218 = And(x=w424, y=w418) -> (x .and. y?=w426:bool)
        n219 = case shown="True" w426 {
          tunnel: w435 -> [_ w489]
          tunnel: w399 -> [_ w488]
          tunnel: w400 -> [_ w487]
          tunnel: w434 -> [_ w486]
          tunnel: w423 -> [_ w485]
          tunnel: w422 -> [_ w484]
          tunnel: w421 -> [_ w483]
          tunnel: w420 -> [_ w482]
          tunnel: 0 ("DMA buffer timeout") -> [_ w491]
          frame False {
          }
          frame True {
            n220 = Build Array(w489, w488, w487, w486, w485, w484, w483, w482) -> (w490:void[])
            n221 = for {
              tunnel: w490 -> [w493] mode=indexing
              tunnel: w491 -> [w494]
              tunnel: [w492] -> w480 mode=indexing
              n222 = xnode ("FIFO Write")("Element"=w493, "Timeout"=w494) -> ("Timed Out?"=w492:bool)  [unwired: 1 in, 1 out]
            }
            n223 = Or Array Elements(Boolean array=w480) -> (logical OR=w477:bool)
            n224 = Boolean To (0,1)(Boolean=w477) -> (0, 1=w479:i16)
            n225 = feedback #23(u16 0) -> (w478:u16)
            n226 = Add(x=w479, y=w478) -> (x+y=w476:u16)
            "Trap AI FIFO Timeout" <- w476
            n227 = feedback-in #23(w476) -> ()
          }
        }
        n228 = feedback-in #21(w402) -> ()
        n229 = feedback-in #22(w418) -> ()
        n230 = case shown="True" w383 {
          tunnel: w382 -> [_ w441]
          tunnel: [u8 0 w438] -> w381
          frame False {
          }
          frame True {
            n231 = Split Number(x=w441) -> (hi(x)=w442:u32, lo(x)=w443:u32)
            n232 = Split Number(x=w442) -> (lo(x)=w444:u16)  [unwired: 1 out]
            n233 = Split Number(x=w443) -> (hi(x)=w445:u16, lo(x)=w446:u16)
            n234 = Build Array "BD 1 nu Stack"(w444, w445, w446) -> (w440:u16[])
            n235 = for {
              tunnel: w440 -> [w453] mode=indexing
              shift-right: [w449] -> w438
              shift-left: u8 0 -> [w450]
              n236 = xnode ("FIFO Method Node")("Element"=w453, "Timeout"="Trap FIFO Set Timeout") -> ("Timed Out?"=w452:bool)  [unwired: 1 in, 1 out]
              n237 = Boolean To (0,1)(Boolean=w452) -> (0, 1=w451:i16)
              n238 = To Unsigned Byte Integer(number=w451) -> (unsigned 8bit integer=w448:u8)
              n239 = Add(x=w448, y=w450) -> (x+y=w449:u8)
            }
          }
        }
        n240 = To Unsigned Word Integer(number=w381) -> (unsigned 16bit integer=w380:u16)
        n241 = feedback #24(u16 0) -> (w394:u16)
        n242 = Add(x=w380, y=w394) -> (x+y=w393:u16)
        "Trap Pos FIFO Timeout" <- w393
        n243 = feedback-in #24(w393) -> ()
        n244 = feedback-in #25(w417) -> ()
        n245 = feedback #25(w417) -> (w416:u16)
        n246 = Subtract(x=w417, y=w416) -> (x-y=w415:u16)
        n247 = xnode "FPGA I/O Node"("Connector1/DIO31"=FALSE ("Connector1/DIO34")) -> ()  [unwired: 1 in, 1 out]
        n248 = Subtract(x=w415, y=w414) -> (x-y=w385:u16)
        n249 = Boolean To (0,1)(Boolean="+ phase") -> (0, 1=w410:i16)
        n250 = Multiply(x=w410, y="Phase count adjustment") -> (x*y=w404:i16)
        n251 = Subtract(x="ai count", y=w385) -> (x-y=w408:u16)
        n252 = Number To Boolean Array(number=w385) -> (Boolean array=w386:bool[])
        n253 = feedback #26(i16 0) -> (w406:i16)
        n254 = Add(x=w408, y=w404) -> (x+y=w407:u16)
        n255 = Subtract(x=w406, y=w404) -> (x-y=w405:i16)
        "Relative phase" <- w405
        n256 = feedback-in #26(w405) -> ()
        n257 = Or Array Elements(Boolean array=w386) -> (logical OR=w384:bool)
        n258 = Boolean To (0,1)(Boolean=w384) -> (0, 1=w391:i16)
        n259 = To Unsigned Byte Integer(number=w391) -> (unsigned 8bit integer=w388:u8)
        n260 = feedback #27(u8 0) -> (w389:u8)
        n261 = Add(x=w388, y=w389) -> (x+y=w387:u8)
        "AI Late Counter" <- w387
        n262 = feedback-in #27(w387) -> ()
      }
    }
  }
  n263 = while "MCL stage control" {
    shift-right: [w510] -> _
    shift-left: w3 -> [w513]
    shift-right: [w503] -> _
    shift-left: w8 -> [w500]
    shift-right: [w502] -> _
    shift-left: w7 -> [w498]
    i -> [w497]
    stop <- FALSE stop-if-true
    n264 = flat-sequence {
      tunnel: w513 -> [w517]
      tunnel: [w518] -> w509
      tunnel: [w517] -> w507
      tunnel: [w516] -> w501
      tunnel: w500 -> [w516]
      tunnel: [w515] -> w499
      tunnel: w498 -> [w515]
      tunnel: w509 -> [w522]
      tunnel: [w522] -> w508
      tunnel: w507 -> [w521]
      tunnel: [w521] -> w506
      tunnel: w501 -> [w520]
      tunnel: w499 -> [w519]
      tunnel: [w520] -> w496
      tunnel: [w519] -> w495
      tunnel: w508 -> [w532]
      tunnel: w506 -> [w531]
      tunnel: [w532] -> w512
      tunnel: [w531] -> w511
      tunnel: [w530] -> w505
      tunnel: [w529] -> w504
      tunnel: w496 -> [w524]
      tunnel: w495 -> [w523]
      tunnel: [w604] -> w510
      tunnel: w512 -> [w611]
      tunnel: w511 -> [w608]
      tunnel: w505 -> [w606]
      tunnel: w504 -> [w605]
      tunnel: [w606] -> w503
      tunnel: [w605] -> w502
      frame #0 {
        n265 = call "Loop Timer5"("Count(Ticks)"=w517) -> ("Tick Count(Ticks)"=w518:u32)
      }
      frame #1 {
        n266 = xnode "FPGA I/O Node"("Connector0/AO1"=w520, "Connector0/AO2"=w519) -> ()  [unwired: 2 in, 2 out]
      }
      frame #2 {
        n267 = local read "Scanning MCL"() -> (w544:bool)
        n268 = Or(x=w544, y="Start scan (MCL)") -> (x .or. y?=w539:bool)
        n269 = Not(x="Abort scan (MCL)") -> (.not. x?=w537:bool)
        n270 = And(x=w537, y=w539) -> (x .and. y?=w536:bool)
        n271 = case "Raster scan" shown="True" w536 {
          tunnel: [w545 w588] -> w541
          tunnel: "Start scan (MCL)" -> [_ w573]
          tunnel: [w545 w549] -> w525
          frame False {
            w545 = i16 0
            n272 = local write "Scanning MCL"(FALSE ("scanning")) -> ()
          }
          frame True {
            w559 = i16 0
            w558 = u64 0
            # "scan incr."
            # "freq. incr. mult."
            # "count steps"
            # "count number of cycles"
            n273 = feedback #28(w558) -> (w585:u64)
            n274 = Select(t=w558, s=w573, f=w585) -> (s? t:f=w587:u64)
            n275 = Increment(x=w587) -> (x+1=w584:u64)
            n276 = Greater?(x="Cycles per step (MCL)", y=w584) -> (0:w568:bool)
            n277 = Select(t=w584, s=w568, f=w558) -> (s? t:f=w583:u64)
            n278 = feedback-in #28(w583) -> ()
            n279 = feedback #29(w558) -> (w582:u64)
            n280 = Select(t=w558, s=w573, f=w582) -> (s? t:f=w577:u64)
            n281 = Increment(x=w577) -> (x+1=w581:u64)
            n282 = Add(x="Scan steps (MCL)", y="Scan steps (MCL)") -> (x+y=w580:u64)
            n283 = Select(t=w577, s=w568, f=w581) -> (s? t:f=w563:u64)
            n284 = Greater?(x=w580, y=w563) -> (0:w562:bool)
            n285 = Select(t=w563, s=w562, f=w558) -> (s? t:f=w578:u64)
            n286 = feedback-in #29(w578) -> ()
            n287 = Equal?(x="Scan steps (MCL)", y=w563) -> (x = y?=w567:bool)
            n288 = Greater?(x="Scan steps (MCL)", y=w577) -> (0:w576:bool)
            n289 = feedback #30(w559) -> (w579:i16)
            n290 = Select(t=w559, s=w573, f=w579) -> (s? t:f=w565:i16)
            n291 = Increment(x=w565) -> (x+1=w575:i16)
            n292 = Decrement(x=w565) -> (x-1=w574:i16)
            n293 = Select(t=w575, s=w576, f=w574) -> (s? t:f=w566:i16)
            n294 = Select(t=w565, s=w567, f=w566) -> (s? t:f=w564:i16)
            n295 = Select(t=w565, s=w568, f=w564) -> (s? t:f=w560:i16)
            n296 = Select(t=w560, s=w562, f=w559) -> (s? t:f=w561:i16)
            n297 = feedback-in #30(w561) -> ()
            n298 = feedback #31(w558) -> (w572:u64)
            n299 = Select(t=w558, s=w573, f=w572) -> (s? t:f=w547:u64)
            n300 = Increment(x=w547) -> (x+1=w569:u64)
            n301 = Select(t=w547, s=w562, f=w569) -> (s? t:f=w548:u64)
            n302 = Greater?(x="Number of scans (MCL)", y=w548) -> (0:w555:bool)
            n303 = Multiply(x="Scan freq.  increment (MCL)", y=w565) -> (x*y=w588:i16)
            n304 = Select(t=TRUE, s="Cont. Scan (MCL)", f=w555) -> (s? t:f=w554:bool)
            "Scanning MCL" <- w554
            n305 = Select(t=w548, s=w554, f=w558) -> (s? t:f=w570:u64)
            n306 = feedback-in #31(w570) -> ()
            n307 = Increment(x=w548) -> (x+1=→"Scan I (MCL)":u64)
            n308 = To Word Integer(number=w547) -> (16bit integer=w550:i16)
            n309 = Multiply(x=w550, y="Scan freq.  increment (MCL)") -> (x*y=w549:i16)
          }
        }
        n310 = Select(t=w525, s="1D or 2D Scan?", f=i16 0) -> (s? t:f=w526:i16)
        n311 = Select(t=w526, s="MCL Scan Axis", f=w541) -> (s? t:f=w540:i16)
        n312 = Select(t=w541, s="MCL Scan Axis", f=w526) -> (s? t:f=w542:i16)
        n313 = Add(x=w540, y="AO2") -> (x+y=w529:i16)
        n314 = Add(x="AO1", y=w542) -> (x+y=w530:i16)
        "AO1 2" <- w524
        "AO2 2" <- w523
      }
      frame #3 {
        n315 = feedback-in #32(w611) -> ()
        n316 = feedback #32(w611) -> (w610:u32)
        n317 = Boolean To (0,1)(Boolean="+ phase (MCL)") -> (0, 1=w602:i16)
        n318 = Subtract(x=w611, y=w610) -> (x-y=w609:u32)
        n319 = Multiply(x=w602, y="Phase count adjustment (MCL)") -> (x*y=w598:i16)
        n320 = Subtract(x=w609, y=w608) -> (x-y=w590:u32)
        n321 = Subtract(x="MCL count", y=w590) -> (x-y=w600:u32)
        n322 = feedback #33(i16 0) -> (w599:i16)
        n323 = Subtract(x=w599, y=w598) -> (x-y=w597:i16)
        "MCL Relative Phase" <- w597
        n324 = feedback-in #33(w597) -> ()
        n325 = Number To Boolean Array(number=w590) -> (Boolean array=w591:bool[])
        n326 = Or Array Elements(Boolean array=w591) -> (logical OR=w589:bool)
        n327 = Boolean To (0,1)(Boolean=w589) -> (0, 1=w596:i16)
        n328 = Add(x=w600, y=w598) -> (x+y=w604:u32)
        n329 = To Unsigned Byte Integer(number=w596) -> (unsigned 8bit integer=w593:u8)
        n330 = feedback #34(u8 0) -> (w594:u8)
        n331 = Add(x=w593, y=w594) -> (x+y=w592:u8)
        "MCL Late Counter" <- w592
        n332 = feedback-in #34(w592) -> ()
      }
    }
    "Numeric" <- w497
  }
  n333 = while "RF box board direct communication loop" {
    tunnel: w3 -> [_]
    stop <- FALSE stop-if-true
    n334 = case "Whether to use direct communication method (only use one method at a time)" shown="True" "Direct RF Box \nCommunication" {
      frame False {
      }
      frame True {
        n335 = case shown="True" "Update Data" {
          frame False {
          }
          frame True {
            n336 = flat-sequence {
              frame #0 {
                n337 = First Call?() -> (First Call?: T/F=w616:bool)
                n338 = case shown="True" w616 {
                  frame False {
                  }
                  frame True {
                    # "If first time data updated, be sure to set WR high\nbefore setting data and address bits."
                    n339 = flat-sequence {
                      frame #0 {
                        n340 = xnode "FPGA I/O Node"("Connector1/DIO15"=TRUE) -> ()  [unwired: 1 in, 1 out]
                      }
                      frame #1 {
                        n341 = call "Wait"("Count(Ticks)"=u8 40 ("DO Delay 3 (Ticks)")) -> ()  [unwired: 1 out]
                      }
                    }
                  }
                }
              }
              frame #1 {
                n342 = Number To Boolean Array(number="Address") -> (Boolean array=w665:bool[])
                n343 = Number To Boolean Array(number="Data BD 1") -> (Boolean array=w666:bool[])
                n344 = Number To Boolean Array(number="Data BD 2") -> (Boolean array=w635:bool[])
                n345 = Index Array(array=w666, index=7) -> (element=w650:bool)
                n346 = Index Array(array=w666, index=6) -> (element=w649:bool)
                n347 = Index Array(array=w666, index=5) -> (element=w648:bool)
                n348 = Index Array(array=w666, index=4) -> (element=w647:bool)
                n349 = Index Array(array=w666, index=3) -> (element=w646:bool)
                n350 = Index Array(array=w666, index=2) -> (element=w645:bool)
                n351 = Index Array(array=w666, index=1) -> (element=w644:bool)
                n352 = Index Array(array=w666, index=0) -> (element=w643:bool)
                n353 = Index Array(array=w665, index=5) -> (element=w642:bool)
                n354 = Index Array(array=w665, index=4) -> (element=w641:bool)
                n355 = Index Array(array=w665, index=3) -> (element=w640:bool)
                n356 = Index Array(array=w665, index=2) -> (element=w639:bool)
                n357 = Index Array(array=w665, index=1) -> (element=w638:bool)
                n358 = Index Array(array=w665, index=0) -> (element=w637:bool)
                n359 = Index Array(array=w635, index=7) -> (element=w626:bool)
                n360 = Index Array(array=w635, index=6) -> (element=w625:bool)
                n361 = Index Array(array=w635, index=5) -> (element=w624:bool)
                n362 = Index Array(array=w635, index=4) -> (element=w623:bool)
                n363 = Index Array(array=w635, index=3) -> (element=w622:bool)
                n364 = Index Array(array=w635, index=2) -> (element=w621:bool)
                n365 = Index Array(array=w635, index=1) -> (element=w620:bool)
                n366 = Index Array(array=w635, index=0) -> (element=w619:bool)
                n367 = xnode "FPGA I/O Node"("Connector1/DIO0"=w650, "Connector1/DIO1"=w649, "Connector1/DIO2"=w648, "Connector1/DIO3"=w647, "Connector1/DIO4"=w646, "Connector1/DIO5"=w645, "Connector1/DIO6"=w644, "Connector1/DIO7"=w643, "Connector1/DIO8"=w642, "Connector1/DIO9"=w641, "Connector1/DIO10"=w640, "Connector1/DIO11"=w639, "Connector1/DIO12"=w638, "Connector1/DIO13"=w637, "Connector1/DIO20"=w626, "Connector1/DIO21"=w625, "Connector1/DIO22"=w624, "Connector1/DIO23"=w623, "Connector1/DIO24"=w622, "Connector1/DIO25"=w621, "Connector1/DIO26"=w620, "Connector1/DIO27"=w619) -> ()  [unwired: 22 in, 22 out]
              }
              frame #2 {
                # "wait and then apply write signal"
                n368 = call "Wait2"("Count(Ticks)"=u8 40 ("DO Delay 1 (Ticks)")) -> ()  [unwired: 1 out]
              }
              frame #3 {
                # "sending bit low writes data to board buffer"
                n369 = xnode "FPGA I/O Node"("Connector1/DIO15"=FALSE) -> ()  [unwired: 1 in, 1 out]
              }
              frame #4 {
                # "wait then return write signal"
                n370 = call "Wait3"("Count(Ticks)"=u8 40 ("DO Delay 2 (Ticks)")) -> ()  [unwired: 1 out]
              }
              frame #5 {
                # "sending bit high makes ready to\nwrite more data"
                n371 = xnode "FPGA I/O Node"("Connector1/DIO15"=TRUE) -> ()  [unwired: 1 in, 1 out]
              }
            }
          }
        }
      }
    }
  }
  n372 = while "Control APD data integration - stream to host" {
    shift-right: [w675] -> _
    shift-left: w3 -> [w680]
    stop <- FALSE stop-if-true
    n373 = flat-sequence {
      tunnel: w680 -> [w682]
      tunnel: [w683] -> w678
      tunnel: [w682] -> w676
      tunnel: [w691] -> w679
      tunnel: w678 -> [w691]
      tunnel: [w690] -> w677
      tunnel: w676 -> [w690]
      tunnel: [w689] -> w674
      tunnel: [w688] -> w673
      tunnel: [w725] -> w675
      tunnel: w679 -> [w737]
      tunnel: w677 -> [w734]
      tunnel: w674 -> [w718]
      tunnel: w673 -> [w717]
      frame #0 {
        n374 = call "Loop Timer6"("Count(Ticks)"=w682) -> ("Tick Count(Ticks)"=w683:u32)
      }
      frame #1 {
        n375 = flat-sequence {
          tunnel: [w693] -> w687
          tunnel: w687 -> [w695]
          tunnel: [w697] -> w686
          tunnel: [w696] -> w685
          tunnel: [w695] -> w684
          tunnel: [w703] -> w688
          tunnel: [w704] -> w689
          tunnel: w686 -> [w704]
          tunnel: w685 -> [w703]
          tunnel: w684 -> [w702]
          frame #0 {
            # "use two separate variable so each APD won't\nhave to wait to read"
            n376 = feedback #35(FALSE) -> (w692:bool)
            "APD 1 out state" <- w692
            "APD 2 out state" <- w692
            n377 = Not(x=w692) -> (.not. x?=w693:bool)
            n378 = feedback-in #35(w693) -> ()
          }
          frame #1 {
            n379 = local read "APD 1 Counts 1"() -> (w701:u32)
            n380 = local read "APD 1 Counts 0"() -> (w700:u32)
            n381 = local read "APD 2 Counts 1"() -> (w699:u32)
            n382 = local read "APD 2 Counts 0"() -> (w698:u32)
            n383 = Select(t=w701, s=w695, f=w700) -> (s? t:f=w697:u32)
            n384 = Select(t=w699, s=w695, f=w698) -> (s? t:f=w696:u32)
          }
          frame #2 {
            n385 = case shown="True" w702 {
              frame False {
                w705 = u32 0 ("APD 1 Counts 0")
                n386 = local write "APD 1 Counts 0"(w705) -> ()
                n387 = local write "APD 2 Counts 0"(w705) -> ()
              }
              frame True {
                w706 = u32 0 ("APD 1 Counts 1")
                n388 = local write "APD 1 Counts 1"(w706) -> ()
                n389 = local write "APD 2 Counts 1"(w706) -> ()
              }
            }
          }
        }
      }
      frame #2 {
        n390 = feedback-in #36(w737) -> ()
        n391 = feedback #36(w737) -> (w736:u32)
        n392 = Subtract(x=w737, y=w736) -> (x-y=w735:u32)
        n393 = Subtract(x=w735, y=w734) -> (x-y=w710:u32)
        n394 = case shown="True" "APD to FIFO" {
          tunnel: w718 -> [_ w740]
          tunnel: w717 -> [_ w738]
          frame False {
          }
          frame True {
            n395 = flat-sequence {
              tunnel: 0 ("Timeout") -> [w742]
              tunnel: w740 -> [w743]
              tunnel: [w742] -> w739
              tunnel: w739 -> [w745]
              tunnel: w738 -> [w744]
              frame #0 {
                n396 = xnode ("FIFO Write")("Element"=w743, "Timeout"=w742) -> ()  [unwired: 1 in, 2 out]
              }
              frame #1 {
                n397 = xnode ("FIFO Write")("Element"=w744, "Timeout"=w745) -> ()  [unwired: 1 in, 2 out]
              }
            }
          }
        }
        n398 = Subtract(x="APD Acq Rate Count", y=w710) -> (x-y=w726:u32)
        n399 = Number To Boolean Array(number=w710) -> (Boolean array=w711:bool[])
        n400 = Or Array Elements(Boolean array=w711) -> (logical OR=w709:bool)
        n401 = Boolean To (0,1)(Boolean=w709) -> (0, 1=w716:i16)
        n402 = To Unsigned Byte Integer(number=w716) -> (unsigned 8bit integer=w713:u8)
        n403 = Boolean To (0,1)(Boolean="+ phase (APD Acq)") -> (0, 1=w722:i16)
        n404 = feedback #37(u8 0) -> (w714:u8)
        n405 = Add(x=w713, y=w714) -> (x+y=w712:u8)
        "APD Acq Late Counter" <- w712
        n406 = feedback-in #37(w712) -> ()
        n407 = Multiply(x=w722, y="Phase Count Adjustment (APD Acq)") -> (x*y=w719:i16)
        n408 = Add(x=w726, y=w719) -> (x+y=w725:u32)
        n409 = feedback #38(i16 0) -> (w724:i16)
        n410 = Subtract(x=w724, y=w719) -> (x-y=w721:i16)
        "APD Acq Relative Phase" <- w721
        n411 = feedback-in #38(w721) -> ()
        n412 = To Word Integer(number=w718) -> (16bit integer=w727:i16)
        n413 = To Word Integer(number=w717) -> (16bit integer=w728:i16)
        n414 = Multiply(x="APD 1 AO scale factor", y=w727) -> (x*y=w708:i16)
        n415 = Multiply(x="APD 2 AO scale factor", y=w728) -> (x*y=w707:i16)
        n416 = xnode "FPGA I/O Node"("Connector0/AO5"=w708, "Connector0/AO7"=w707) -> ()  [unwired: 2 in, 2 out]
      }
    }
  }
  n417 = while "RF box board DIO control: parallel communication" {
    shift-right: [w752] -> _
    shift-left: w3 -> [w751]
    shift-right: [w750] -> _
    shift-left: FALSE ("Swap F1 and F2") -> [w749]
    stop <- FALSE stop-if-true
    n418 = flat-sequence {
      tunnel: w749 -> [w756]
      tunnel: w751 -> [w754]
      tunnel: [w756] -> w748
      tunnel: [w755] -> w747
      tunnel: [w754] -> w746
      tunnel: [w762] -> w752
      tunnel: [w761] -> w750
      tunnel: w748 -> [w760]
      tunnel: w747 -> [w758]
      tunnel: w746 -> [w757]
      frame #0 {
        n419 = call "Loop Timer"("Count(Ticks)"=w754) -> ("Tick Count(Ticks)"=w755:u16)
      }
      frame #1 {
        n420 = flat-sequence {
          tunnel: ["FPGA Controls\n RF Box"] -> w759
          tunnel: w760 -> [w763]
          tunnel: [w803] -> w762
          tunnel: [w816] -> w761
          tunnel: w759 -> [w815]
          tunnel: w758 -> [w809]
          tunnel: w757 -> [w806]
          frame #0 {
            n421 = case shown="True" "FPGA Controls\n RF Box" {
              tunnel: w763 -> [_ w765]
              frame False {
              }
              frame True {
                n422 = flat-sequence {
                  tunnel: w765 -> [w771]
                  frame #0 {
                    n423 = First Call?() -> (First Call?: T/F=w766:bool)
                    n424 = case shown="True" w766 {
                      frame False {
                      }
                      frame True {
                        # "If first time data updated, be sure to set WR high and UDCLK low\nbefore setting data and address bits."
                        n425 = xnode "FPGA I/O Method Node"("Enable"=TRUE) -> ("FPGA I/O Out"=w768:refnum<k21>)  [unwired: 1 in]
                        n426 = xnode "FPGA I/O Node"("Connector1/DIO15"=TRUE) -> ()  [unwired: 1 in, 1 out]
                        n427 = xnode "FPGA I/O Node"("I/O Item"=FALSE ("Connector1/DIO30"), "FPGA I/O In"=w768) -> ()  [unwired: 1 out]
                      }
                    }
                  }
                  frame #1 {
                    n428 = case shown="True" "Freq or Amp switch first" {
                      tunnel: w771 -> [w773 w778]
                      frame False {
                        n429 = flat-sequence {
                          tunnel: w773 -> [w777]
                          frame #0 {
                            # "switch amplitude"
                            # "send udclk high"
                            n430 = xnode "FPGA I/O Node"("Connector1/DIO30"=TRUE ("Connector1/DIO15")) -> ()  [unwired: 1 in, 1 out]
                          }
                          frame #1 {
                            # "send udclk low"
                            n431 = xnode "FPGA I/O Node"("Connector1/DIO30"=FALSE ("Connector1/DIO15")) -> ()  [unwired: 1 in, 1 out]
                          }
                          frame #2 {
                            n432 = call "Wait5"("Count(Ticks)"="Freq switch delay") -> ()  [unwired: 1 out]
                          }
                          frame #3 {
                            # "switch frequency"
                            n433 = xnode "FPGA I/O Node"("Connector1/DIO36"=w777) -> ()  [unwired: 1 in, 1 out]
                          }
                        }
                      }
                      frame True {
                        n434 = flat-sequence {
                          tunnel: w778 -> [w779]
                          frame #0 {
                            # "switch frequency"
                            n435 = xnode "FPGA I/O Node"("Connector1/DIO36"=w779) -> ()  [unwired: 1 in, 1 out]
                          }
                          frame #1 {
                            n436 = call "Wait4"("Count(Ticks)"="Amp switch delay") -> ()  [unwired: 1 out]
                          }
                          frame #2 {
                            # "switch amplitude"
                            # "send udclk high"
                            n437 = xnode "FPGA I/O Node"("Connector1/DIO30"=TRUE ("Connector1/DIO15")) -> ()  [unwired: 1 in, 1 out]
                          }
                          frame #3 {
                            # "send udclk low"
                            n438 = xnode "FPGA I/O Node"("Connector1/DIO30"=FALSE ("Connector1/DIO15")) -> ()  [unwired: 1 in, 1 out]
                          }
                        }
                      }
                    }
                  }
                }
              }
            }
          }
          frame #1 {
            # "This is the prior cycle's on time"
            # "increment timing\nindex, reset to 0 if \nend of matrix"
            # "Reset to begginning (1) when number of cycles reached."
            # "timing index"
            # "build byte stacks for writing data\n(must correspond to addresses array constant)"
            # "Timing housekeeping"
            # "Adjust phase if late\n(maintains constant phase relationship between cycles)"
            n439 = feedback #39(u8 0 ("t")) -> (w812:u8)
            n440 = Increment(x=w812) -> (x+1=w856:u8)
            n441 = Increment(x="Number Interlace Cycles") -> (x+1=w851:u8)
            n442 = Equal?(x=w856, y=w851) -> (x = y?=w858:bool)
            n443 = Select(t=u8 1, s=w858, f=w856) -> (s? t:f=w811:u8)
            n444 = feedback-in #39(w811) -> ()
            n445 = Increment(x=w811) -> (x+1=w853:u8)
            n446 = Equal?(x=w853, y=w851) -> (x = y?=w854:bool)
            n447 = Select(t=u8 1, s=w854, f=w853) -> (s? t:f=w850:u8)
            n448 = Select(t=w850, s="Interlace ON/OFF", f="Interlace Off Parameters") -> (s? t:f=w834:u8)
            n449 = case shown="1, Default" w834 {
              tunnel: [w928 w1093 "BD 1 Frequency 3"] -> w846
              tunnel: [w927 "BD 2 Frequency 2" "BD 2 Frequency 3"] -> w835
              tunnel: ["BD 2 Amplitude 1" "BD 2 Amplitude 2" "BD 2 Amplitude 3"] -> w791
              tunnel: [w917 w1103 "BD 1 Amplitude 3"] -> w794
              frame 1, Default {
                w908 = fxp<+/-,24,9> 0.0 ("AI1 X Set 2")
                w901 = u16 0
                w923 = u64 0 ("f")
                # "This signal integration happens no matter what\nso that correct setpoints can be chosen before \nturning on the FB."
                # "Trap 1"
                n450 = local read "AI1 X Set 2"() -> (w904:fxp<+/-,16,1>)
                n451 = local read "AI1 X Set 1"() -> (w905:fxp<+/-,16,1>)
                n452 = local read "Scanning"() -> (w929:bool)
                n453 = case shown="False" "Diff FB Measurement?" {
                  tunnel: w904 -> [w937 w946]
                  tunnel: w905 -> [w936 w947]
                  tunnel: [w934 w938] -> w906
                  frame False {
                    n454 = Select(t=w936, s="Trap Pos FB Monitor T1 or T2", f=w937) -> (s? t:f=w934:fxp<+/-,16,1>)
                  }
                  frame True {
                    n455 = Subtract(x=w947, y=w946) -> (x-y=w939:fxp<+/-,17,2>)
                    n456 = Not(x="Negate Diff?") -> (.not. x?=w945:bool)
                    n457 = Boolean To (0,1)(Boolean="Negate Diff?") -> (0, 1=w943:i16)
                    n458 = Boolean To (0,1)(Boolean=w945) -> (0, 1=w944:i16)
                    n459 = Negate(x=w943) -> (-x=w942:i16)
                    n460 = Add(x=w942, y=w944) -> (x+y=w940:i16)
                    n461 = Multiply(x=w940, y=w939) -> (x*y=w938:fxp<+/-,32,17>)
                  }
                }
                n462 = Or(x=w929, y="Start scan") -> (x .or. y?=w921:bool)
                n463 = Not(x="Abort scan") -> (.not. x?=w919:bool)
                n464 = And(x=w919, y=w921) -> (x .and. y?=w892:bool)
                n465 = feedback #40(w901) -> (w900:u16)
                n466 = Increment(x=w900) -> (x+1=w902:u16)
                n467 = Greater Or Equal?(x=w902, y="Trap Pos FB Int Count") -> (x >= y?=w893:bool)
                n468 = case "For raster scanning" shown="False" w892 {
                  tunnel: [w1034 w1046] -> w924
                  tunnel: "Start scan" -> [_ w1070]
                  frame False {
                    # "For wiggle-calibration: sinusoidal wave"
                    n469 = local read "Wiggling 1"() -> (w1029:bool)
                    n470 = Not(x="Abort wiggle 1") -> (.not. x?=w1032:bool)
                    n471 = Or(x="Wiggle trap 1", y=w1029) -> (x .or. y?=w1028:bool)
                    n472 = And(x=w1028, y=w1032) -> (x .and. y?=w1031:bool)
                    n473 = case shown="True" w1031 {
                      tunnel: [u64 0 w1042] -> w1034
                      frame False {
                        n474 = local write "Wiggling 1"(FALSE ("Wiggle")) -> ()
                      }
                      frame True {
                        # "Input is periods/tick, not Hz,\nso need to normalize by clock\nfrequency (40 MHz)."
                        n475 = Divide(x="Wiggle freq 1 (Hz)", y=fxp<+,17,26> 40000000.0) -> (x/y=w1039:fxp<+/-,17,-9>)
                        n476 = call "Sine Wave Generator"("frequency (periods/tick)"=w1039) -> ("sine out"=w1044:i32)  [unwired: 14 in]
                        n477 = Multiply(x=w1044, y="Wiggle amp 1") -> (x*y=w1042:u64)
                        "Wiggling 1" <- TRUE
                      }
                    }
                    n478 = local write "Scanning"(FALSE ("scanning")) -> ()
                  }
                  frame True {
                    w1054 = i64 0
                    w1053 = u64 0
                    # "scan incr."
                    # "freq. incr. mult."
                    # "count steps"
                    # "count number of cycles"
                    n479 = feedback #41(w1053) -> (w1082:u64)
                    n480 = Select(t=w1053, s=w1070, f=w1082) -> (s? t:f=w1084:u64)
                    n481 = Increment(x=w1084) -> (x+1=w1081:u64)
                    n482 = Greater?(x="Cycles per step", y=w1081) -> (0:w1063:bool)
                    n483 = Select(t=w1081, s=w1063, f=w1053) -> (s? t:f=w1080:u64)
                    n484 = feedback-in #41(w1080) -> ()
                    n485 = feedback #42(w1053) -> (w1079:u64)
                    n486 = Select(t=w1053, s=w1070, f=w1079) -> (s? t:f=w1074:u64)
                    n487 = Increment(x=w1074) -> (x+1=w1078:u64)
                    n488 = Add(x="Scan steps", y="Scan steps") -> (x+y=w1077:u64)
                    n489 = Select(t=w1074, s=w1063, f=w1078) -> (s? t:f=w1058:u64)
                    n490 = Greater?(x=w1077, y=w1058) -> (0:w1057:bool)
                    n491 = Select(t=w1058, s=w1057, f=w1053) -> (s? t:f=w1075:u64)
                    n492 = feedback-in #42(w1075) -> ()
                    n493 = Equal?(x="Scan steps", y=w1058) -> (x = y?=w1062:bool)
                    n494 = Greater?(x="Scan steps", y=w1074) -> (0:w1073:bool)
                    n495 = feedback #43(w1054) -> (w1076:i64)
                    n496 = Select(t=w1054, s=w1070, f=w1076) -> (s? t:f=w1060:i64)
                    n497 = Increment(x=w1060) -> (x+1=w1072:i64)
                    n498 = Decrement(x=w1060) -> (x-1=w1071:i64)
                    n499 = Select(t=w1072, s=w1073, f=w1071) -> (s? t:f=w1061:i64)
                    n500 = Select(t=w1060, s=w1062, f=w1061) -> (s? t:f=w1059:i64)
                    n501 = Select(t=w1060, s=w1063, f=w1059) -> (s? t:f=w1055:i64)
                    n502 = Select(t=w1055, s=w1057, f=w1054) -> (s? t:f=w1056:i64)
                    n503 = feedback-in #43(w1056) -> ()
                    n504 = feedback #44(w1053) -> (w1069:u64)
                    n505 = Select(t=w1053, s=w1070, f=w1069) -> (s? t:f=w1065:u64)
                    n506 = Increment(x=w1065) -> (x+1=w1066:u64)
                    n507 = Select(t=w1065, s=w1057, f=w1066) -> (s? t:f=w1064:u64)
                    n508 = Greater?(x="Number of scans", y=w1064) -> (0:w1050:bool)
                    n509 = Multiply(x="Scan freq.  increment", y=w1060) -> (x*y=w1046:i64)
                    n510 = Select(t=TRUE, s="Cont. Scan", f=w1050) -> (s? t:f=w1049:bool)
                    "Scanning" <- w1049
                    n511 = Select(t=w1064, s=w1049, f=w1053) -> (s? t:f=w1067:u64)
                    n512 = feedback-in #44(w1067) -> ()
                    n513 = Increment(x=w1064) -> (x+1=→"Scan I":u64)
                  }
                }
                n514 = Select(t=w901, s=w893, f=w902) -> (s? t:f=w903:u16)
                n515 = feedback-in #40(w903) -> ()
                n516 = feedback #45(w908) -> (w907:fxp<+/-,24,9>)
                n517 = Add(x=w906, y=w907) -> (x+y=w899:fxp<+/-,24,9>)
                n518 = Select(t=w908, s=w893, f=w899) -> (s? t:f=w911:fxp<+/-,24,9>)
                n519 = feedback-in #45(w911) -> ()
                n520 = Divide(x=w899, y="Trap Pos FB Int Count") -> (x/y=w894:fxp<+/-,16,1>)
                n521 = feedback #46(fxp<+/-,24,9> 0.0 ("AI1 X Set 2")) -> (w912:fxp<+/-,24,9>)
                n522 = Select(t=w899, s=w893, f=w912) -> (s? t:f=w913:fxp<+/-,24,9>)
                "Trap Pos FB Int Signal" <- w913
                n523 = feedback-in #46(w913) -> ()
                n524 = feedback #47(fxp<+/-,16,1> 0.0 ("Trap Pos FB Int-Norm Signal")) -> (w896:fxp<+/-,16,1>)
                n525 = Select(t=w894, s=w893, f=w896) -> (s? t:f=w895:fxp<+/-,16,1>)
                "Trap Pos FB Int-Norm Signal" <- w895
                n526 = feedback-in #47(w895) -> ()
                n527 = case "For position feedback" shown="True" "Force feedback" {
                  tunnel: [i64 0 w953] -> w914
                  tunnel: w894 -> [_ w950]
                  tunnel: w893 -> [_ w949]
                  frame False {
                  }
                  frame True {
                    n528 = feedback #48(i64 0) -> (w952:i64)
                    n529 = case shown="True" w949 {
                      tunnel: [w954 w961] -> w953
                      tunnel: w952 -> [w954 _]
                      tunnel: w950 -> [_ w955]
                      frame False {
                      }
                      frame True {
                        w965 = u32 0
                        n530 = xnode ("PID")("process variable"=w955, "reset?"="Trap Pos. FB Reset", "setpoint"="Trap Pos. FB SP", "PID gains"="Trap Pos. FB Gains", "output range"="Trap Pos. FB Range") -> ("output"=w977:fxp<+/-,16,1>)
                        n531 = Negate(x=w977) -> (-x=w976:fxp<+/-,17,2>)
                        n532 = Select(t=w976, s="Trap Pos FB Negate Action", f=w977) -> (s? t:f=w973:fxp<+/-,17,2>)
                        n533 = Scale By Power Of 2(n=u32 15, x=u32 1) -> (x*2^n=w970:u32)
                        n534 = Multiply(x=w973, y=w970) -> (x*y=w969:fxp<+/-,17,17>)
                        n535 = To Quad Integer(1:w969) -> (0:w981:i64)
                        "Trap Pos FB Action" <- w981
                        n536 = Multiply(x=w981, y="Trap Pos. FB Mult Factor") -> (x*y=w979:i64)
                        n537 = Add(x=w979, y="Trap Pos. FB Offset Factor") -> (x+y=w961:i64)
                        n538 = feedback #49() -> (w962:i64)  [unwired: 1 in]
                        n539 = Add(x=w961, y=w962) -> (x+y=w959:i64)
                        n540 = feedback #50(w965) -> (w967:u32)
                        n541 = Increment(x=w967) -> (x+1=w956:u32)
                        n542 = Greater Or Equal?(x=w956, y="FB Trig Integrate") -> (x >= y?=w957:bool)
                        n543 = Select(t=i64 0, s=w957, f=w959) -> (s? t:f=w963:i64)
                        n544 = feedback-in #49(w963) -> ()
                        n545 = Select(t=w965, s=w957, f=w956) -> (s? t:f=w966:u32)
                        n546 = feedback-in #50(w966) -> ()
                        n547 = And(x=w957, y="FPGA Trap Trig") -> (x .and. y?=w964:bool)
                        n548 = case "Trap FB trigger excitation laser ON" shown="True" w964 {
                          tunnel: w959 -> [_ w987]
                          tunnel: w956 -> [_ w985]
                          frame False {
                          }
                          frame True {
                            n549 = Not(x="TTrig Negate Pos") -> (.not. x?=w994:bool)
                            n550 = Boolean To (0,1)(Boolean="TTrig Negate Pos") -> (0, 1=w992:i16)
                            n551 = Boolean To (0,1)(Boolean=w994) -> (0, 1=w993:i16)
                            n552 = Negate(x=w992) -> (-x=w991:i16)
                            n553 = Add(x=w991, y=w993) -> (x+y=w990:i16)
                            n554 = Multiply(x=w990, y=w987) -> (x*y=w989:i64)
                            "TTrig Sig" <- w989
                            n555 = Multiply(x="FPGA TTrig Thresh", y=w985) -> (x*y=w986:i64)
                            "TTrig Fin Thresh" <- w986
                            n556 = Greater Or Equal?(x=w989, y=w986) -> (x >= y?=w988:bool)
                            n557 = case shown="True" w988 {
                              frame False {
                              }
                              frame True {
                                w997 = TRUE ("Green FB On/Off")
                                w999 = u8 2 ("Operating Mode")
                                n558 = local write "Operating Mode 2"(w999) -> ()
                                n559 = local write "Operating Mode"(w999) -> ()
                                n560 = local write "Green FB On/Off"(w997) -> ()
                                n561 = local write "FPGA Trap Trig"(FALSE ("FPGA Trap Trig")) -> ()
                                "TTrig?" <- w997
                              }
                            }
                          }
                        }
                      }
                    }
                    n562 = feedback-in #48(w953) -> ()
                  }
                }
                n563 = case "For intensity feedback" shown="True" "FB On/Off Set 1" {
                  tunnel: "BD 1 Amplitude 1" -> [w1085 _]
                  tunnel: [w1085 w1086] -> w917
                  frame False {
                  }
                  frame True {
                    n564 = local read "AI2 Y Sum Set 1"() -> (w1088:i16)
                    n565 = call "Slower PID.vi"("process variable"=w1088, "reset?"="FB Reset Set 1", "setpoint"="FB Setpoint Set 1", "PID gains (x 2^8)"="FB Gains Set 1", "output range"="FB output range 1") -> ("output"=w1091:i16)  [unwired: 10 out]
                    n566 = To Unsigned Word Integer(number=w1091) -> (unsigned 16bit integer=w1086:u16)
                  }
                }
                n567 = Select(t=w923, s="Scan BD", f=w924) -> (s? t:f=w922:u64)
                n568 = Select(t=w924, s="Scan BD", f=w923) -> (s? t:f=w925:u64)
                n569 = Add(x=w922, y="BD 2 Frequency 1") -> (x+y=w927:u64)
                n570 = Compound Arithmetic op=ADD("BD 1 Frequency 1", w914, w925) -> (w928:u64)
                "BD1 Frequency Out 1" <- w928
              }
              frame 2 {
                # "For wiggle calibration"
                # "Trap 2"
                n571 = local read "Wiggling 2"() -> (w1100:bool)
                n572 = Or(x="Wiggle trap 2", y=w1100) -> (x .or. y?=w1099:bool)
                n573 = Not(x="Abort wiggle 2") -> (.not. x?=w1097:bool)
                n574 = And(x=w1099, y=w1097) -> (x .and. y?=w1096:bool)
                n575 = case shown="True" "FB On/Off Set 2" {
                  tunnel: [w1116 w1117] -> w1103
                  tunnel: "BD 1 Amplitude 2" -> [w1116 _]
                  frame False {
                  }
                  frame True {
                    n576 = local read "AI2 Y Sum Set 2"() -> (w1122:i16)
                    n577 = call "Slower PID.vi"("process variable"=w1122, "reset?"="FB Reset Set 2", "setpoint"="FB Setpoint Set 2", "PID gains (x 2^8)"="FB Gains Set 2", "output range"="FB output range 2") -> ("output"=w1119:i16)  [unwired: 10 out]
                    n578 = To Unsigned Word Integer(number=w1119) -> (unsigned 16bit integer=w1117:u16)
                  }
                }
                n579 = case shown="True" w1096 {
                  tunnel: [i16 0 w1110] -> w1094
                  frame False {
                    n580 = local write "Wiggling 2"(FALSE) -> ()
                  }
                  frame True {
                    n581 = Divide(x="Wiggle freq 2 (Hz)", y=fxp<+,17,26> 40000000.0) -> (x/y=w1113:fxp<+/-,17,-9>)
                    n582 = call "Sine Wave Generator2"("frequency (periods/tick)"=w1113) -> ("sine out"=w1112:i32)  [unwired: 14 in]
                    n583 = Multiply(x=w1112, y="Wiggle amp 2") -> (x*y=w1110:u64)
                    "Wiggling 2" <- TRUE
                  }
                }
                n584 = Add(x="BD 1 Frequency 2", y=w1094) -> (x+y=w1093:u64)
                "BD1 Frequency Out 2" <- w1093
              }
              frame 3 {
                # "Fluorescence period"
              }
            }
            n585 = feedback-in #51(w809) -> ()
            n586 = feedback #51(w809) -> (w808:u16)
            n587 = Select(t=w811, s="Interlace ON/OFF", f="Interlace Off Parameters") -> (s? t:f=w849:u8)
            n588 = Subtract(x=w809, y=w808) -> (x-y=w807:u16)
            n589 = Subtract "The error"(x=w807, y=w806) -> (x-y=w784:u16)
            n590 = case shown="3" w849 {
              tunnel: ["DIO count 1 (ticks)" "DIO count 2 (ticks)" "DIO count 3 (ticks)"] -> w805
              frame 1, Default {
              }
              frame 2 {
              }
              frame 3 {
              }
            }
            n591 = Number To Boolean Array(number=w784) -> (Boolean array=w785:bool[])
            n592 = Or Array Elements(Boolean array=w785) -> (logical OR=w783:bool)
            n593 = Boolean To (0,1)(Boolean=w783) -> (0, 1=w790:i16)
            n594 = To Unsigned Byte Integer(number=w790) -> (unsigned 8bit integer=w787:u8)
            n595 = feedback #52(u8 0) -> (w788:u8)
            n596 = Add(x=w787, y=w788) -> (x+y=w786:u8)
            "DIO Late Counter" <- w786
            n597 = feedback-in #52(w786) -> ()
            n598 = Subtract(x=w805, y=w784) -> (x-y=w804:u16)
            n599 = Split Number(x=w846) -> (hi(x)=w845:u32, lo(x)=w844:u32)
            n600 = Split Number(x=w835) -> (hi(x)=w840:u32, lo(x)=w839:u32)
            n601 = Boolean To (0,1)(Boolean="+ phase (DIO)") -> (0, 1=w801:i16)
            n602 = Split Number(x=w845) -> (lo(x)=w843:u16)  [unwired: 1 out]
            n603 = Split Number(x=w844) -> (hi(x)=w842:u16, lo(x)=w841:u16)
            n604 = Split Number(x=w840) -> (lo(x)=w838:u16)  [unwired: 1 out]
            n605 = Split Number(x=w839) -> (hi(x)=w837:u16, lo(x)=w836:u16)
            n606 = Split Number(x=w794) -> (hi(x)=w796:u8, lo(x)=w795:u8)
            n607 = Split Number(x=w791) -> (hi(x)=w793:u8, lo(x)=w792:u8)
            n608 = Split Number(x=w843) -> (hi(x)=w833:u8, lo(x)=w832:u8)
            n609 = Split Number(x=w842) -> (hi(x)=w831:u8, lo(x)=w830:u8)
            n610 = Split Number(x=w838) -> (hi(x)=w826:u8, lo(x)=w825:u8)
            n611 = Split Number(x=w841) -> (hi(x)=w829:u8, lo(x)=w828:u8)
            n612 = Split Number(x=w837) -> (hi(x)=w824:u8, lo(x)=w823:u8)
            n613 = Split Number(x=w836) -> (hi(x)=w822:u8, lo(x)=w821:u8)
            n614 = Multiply(x=w801, y="Phase count adjustment (DIO)") -> (x*y=w797:i16)
            n615 = feedback #53(i16 0) -> (w799:i16)
            n616 = Subtract(x=w799, y=w797) -> (x-y=w798:i16)
            "DIO Relative phase" <- w798
            n617 = feedback-in #53(w798) -> ()
            n618 = Add(x=w804, y=w797) -> (x+y=w803:u16)
            n619 = Build Array "BD 1 A Stack"(w796, w795) -> (w818:u8[])
            n620 = Build Array "BD 2 A Stack"(w793, w792) -> (w817:u8[])
            n621 = Build Array "BD 1 nu Stack"(w833, w832, w831, w830, w829, w828) -> (w827:u8[])
            n622 = Build Array "BD 2 nu Stack"(w826, w825, w824, w823, w822, w821) -> (w820:u8[])
            n623 = case shown="2" w834 {
              tunnel: [w884 w887] -> w816
              tunnel: [u8 10 u8 4] -> w819
              tunnel: "Swap F1 and F2" -> [w885 w887]
              frame 2 {
                # "F2"
                n624 = Not(x=w885) -> (.not. x?=w884:bool)
              }
              frame 1, Default {
                # "low chooses F1"
                # "F1"
              }
            }
            n625 = case "If FPGA is controlling (toggling) RF synth" shown="True" w815 {
              tunnel: w827 -> [_ w863]
              tunnel: w820 -> [_ w862]
              tunnel: w819 -> [_ w861]
              tunnel: w818 -> [_ w860]
              tunnel: w817 -> [_ w859]
              frame False {
              }
              frame True {
                # "Write next amp.\n(wait until beginning of next loop iteration to update)"
                n626 = flat-sequence "Update the next F1 and F2 frequency value (the actual frequency won't change until FSK is switched).\nThen load the next amplitude value into buffer, but don't update it until the next cycle." {
                  tunnel: w863 -> [w866]
                  tunnel: w862 -> [w865]
                  tunnel: w861 -> [w864]
                  tunnel: w860 -> [w877]
                  tunnel: w859 -> [w876]
                  frame #0 {
                    n627 = for {
                      tunnel: w866 -> [w872] mode=indexing
                      tunnel: w865 -> [w871] mode=indexing
                      tunnel: w864 -> [w869]
                      i -> [w870]
                      # "Write next freq."
                      n628 = To Unsigned Byte Integer(number=w870) -> (unsigned 8bit integer=w867:u8)
                      n629 = Add(x=w869, y=w867) -> (x+y=w868:u8)
                      n630 = call "write to RF synth bd.vi"("Address Byte"=w868, "BD 2 Byte"=w871, "BD 1 Byte"=w872) -> ()
                    }
                  }
                  frame #1 {
                    # "send udclk high"
                    n631 = xnode "FPGA I/O Node"("Connector1/DIO30"=TRUE ("Connector1/DIO15")) -> ()  [unwired: 1 in, 1 out]
                  }
                  frame #2 {
                    n632 = xnode "FPGA I/O Node"("Connector1/DIO30"=FALSE ("Connector1/DIO15")) -> ()  [unwired: 1 in, 1 out]
                  }
                  frame #3 {
                    n633 = for {
                      tunnel: w877 -> [w883] mode=indexing
                      tunnel: w876 -> [w882] mode=indexing
                      tunnel: u8 33 -> [w880]
                      i -> [w881]
                      n634 = To Unsigned Byte Integer(number=w881) -> (unsigned 8bit integer=w878:u8)
                      n635 = Add(x=w880, y=w878) -> (x+y=w879:u8)
                      n636 = call "write to RF synth bd.vi"("Address Byte"=w879, "BD 2 Byte"=w882, "BD 1 Byte"=w883) -> ()
                    }
                  }
                }
              }
            }
          }
        }
      }
    }
  }
  n637 = node-c288(w5) -> ()
  n638 = while {
    shift-right: [w1133] -> _
    shift-left: w2 -> [w1135]
    shift-right: [w1128] -> _
    shift-left: w3 -> [w1137]
    stop <- FALSE stop-if-true
    n639 = flat-sequence {
      tunnel: w1137 -> [w1138]
      tunnel: [w1140] -> w1136
      tunnel: w1135 -> [w1140]
      tunnel: [w1139] -> w1131
      tunnel: [w1138] -> w1129
      tunnel: w1136 -> [w1143]
      tunnel: [w1142] -> w1132
      tunnel: w1131 -> [w1142]
      tunnel: [w1141] -> w1130
      tunnel: w1129 -> [w1141]
      tunnel: [w1171] -> w1133
      tunnel: w1132 -> [w1161]
      tunnel: w1130 -> [w1160]
      tunnel: [w1144] -> w1128
      frame #0 {
        n640 = call "Loop Timer11"("Count(Ticks)"=w1138) -> ("Tick Count(Ticks)"=w1139:u16)
      }
      frame #1 {
        n641 = xnode "FPGA I/O Node"("Connector1/DIO32"=w1143, "Connector1/DIO33"=w1143, "Connector1/DIO34"=w1143) -> ()  [unwired: 3 in, 3 out]
      }
      frame #2 {
        n642 = feedback #54(w1161) -> (w1170:u16)
        n643 = feedback-in #54(w1161) -> ()
        n644 = Subtract(x=w1161, y=w1170) -> (x-y=w1169:u16)
        n645 = Subtract(x=w1169, y=w1160) -> (x-y=w1156:u16)
        n646 = Number To Boolean Array(number=w1156) -> (Boolean array=w1163:bool[])
        n647 = Boolean To (0,1)(Boolean="+ phase (RI)") -> (0, 1=w1154:i16)
        n648 = Or Array Elements(Boolean array=w1163) -> (logical OR=w1162:bool)
        n649 = Multiply(x=w1154, y="Phase count adjustment (RI)") -> (x*y=w1152:i16)
        n650 = Boolean To (0,1)(Boolean=w1162) -> (0, 1=w1168:i16)
        n651 = feedback #55(i16 0) -> (w1153:i16)
        n652 = Subtract(x=w1153, y=w1152) -> (x-y=w1151:i16)
        "RI relative phase" <- w1151
        n653 = feedback-in #55(w1151) -> ()
        n654 = To Unsigned Byte Integer(number=w1168) -> (unsigned 8bit integer=w1165:u8)
        n655 = feedback #56(u8 0) -> (w1166:u8)
        n656 = Add(x=w1165, y=w1166) -> (x+y=w1164:u8)
        "RI late counter" <- w1164
        n657 = feedback-in #56(w1164) -> ()
        n658 = feedback #57(TRUE) -> (w1145:bool)
        n659 = case shown="2" "Red operating mode" {
          tunnel: [TRUE FALSE w1175] -> w1171
          tunnel: w1145 -> [_ _ w1177]
          frame 0, Default {
          }
          frame 1 {
          }
          frame 2 {
            n660 = Not(x=w1177) -> (.not. x?=w1176:bool)
            n661 = Select(t=w1176, s="Invert RI", f=w1177) -> (s? t:f=w1175:bool)
          }
        }
        n662 = Not(x=w1145) -> (.not. x?=w1146:bool)
        n663 = Select(t="RI ON count", s=w1146, f="RI OFF count") -> (s? t:f=w1157:u16)
        n664 = Subtract(x=w1157, y=w1156) -> (x-y=w1150:u16)
        n665 = Add(x=w1150, y=w1152) -> (x+y=w1144:u16)
        n666 = feedback-in #57(w1146) -> ()
      }
    }
  }
